vi "ScanCtrl_HRNoFP.vi"() -> ()   [LabVIEW 2020]
uses:
  <vilib>/event_ctls.llb/usereventprio.ctl
  C:/Users/MarcuLab/Desktop/V6 APD LV/V6 APD LV/Kinesis/Thorlabs.MotionControl.KCube.BrushlessMotorCLI.dll
  Kinesis/Thorlabs.MotionControl.KCube.BrushlessMotorCLI.dll
  C:/Users/MarcuLab/Desktop/V6 APD LV/V6 APD LV/Kinesis/ThorLabs.MotionControl.KCube.DCServoCLI.dll
  Kinesis/ThorLabs.MotionControl.KCube.DCServoCLI.dll
  C:/Users/MarcuLab/Desktop/V6 APD LV/V6 APD LV/Kinesis/Thorlabs.MotionControl.DeviceManagerCLI.dll
  Kinesis/Thorlabs.MotionControl.DeviceManagerCLI.dll
  C:/Users/MarcuLab/Desktop/V6 APD LV/V6 APD LV/Kinesis/Thorlabs.MotionControl.GenericMotorCLI.dll
  Kinesis/Thorlabs.MotionControl.GenericMotorCLI.dll
  <userlib>/_OpenG.lib/time/time.llb/openg_time.lvlib
panel:
  in  "GoToScanStart":bool
  in  "Home Button(fast)":bool
  out "Scan Progress":dbl(slide) scale=0.0..100.0
  in  "Jog Step (mm)":dbl=0.5
  in  "Down(Slow)":bool
  in  "Up(Slow)":bool
  in  "Down(Fast)":bool
  in  "Up(Fast)":bool
  out "SlowAxisStatus":T1
  out "SlowAxisInfo":T2
  out "FastAxisStatus":T1
  out "Current State":string
  out "FastAxisInfo":T3
  out "error out":errorcluster
  out "TriggerPara":T4
  out "Trigger1Polarity":i32(ring)=1 items=["TriggerHigh"=1, "TriggerLow"=2]
  out "Trigger1Mode":i32(ring) items=["Disabled"=0, "TrigIN_GPI"=1, "TrigIN_RelativeMove"=2, "TrigIN_AbsoluteMove"=3, "TrigIN_Homed"=4, "TrigIN_Stop"=5, "TrigOUT_GPO"=10, "TrigOUT_InMotion"=11, "TrigOUT_AtMaxVelocity"=12, "TrigOUT_AtPositionFwd"=13, "TrigOUT_AtPositionRev"=14, "TrigOUT_AtPositionBoth"=15, "TrigOut_AtFwdLimit"=16, "TrigOut_AtBwdLimit"=17, "TrigOut_AtLimit"=18]
  in  "acceleration (mm/s2)":dbl=4000.0
  out "ScanRoute":cluster{dbl[], dbl[]}(graph)
  out "# of lines":u32
  in  "Start Scan":bool
  in  "Comp Scan Para":bool
  out "X speed (mm/s)":dbl format="%.4g"
  in  "Laser Rate (Hz)":u16=2500
  in  "Y step size (um)":dbl=50.0
  in  "X step size (um)":dbl=10.0
  in  "Y scan distance (mm)":dbl=15.0
  in  "X scan distance (mm)":dbl=15.0
  out "Y0 Position(mm)":dbl format="%.4g"
  out "GetPositionCounter 2":i32
  out "X0 Position(mm)":dbl format="%.4g"
  out "GetPositionCounter":i32
  in  "SetScanStart":bool
  in  "SerialNumber(Slow)":string="27000986"
  in  "SerialNumber(Fast)":string="28252795"
  in  "Quit":bool
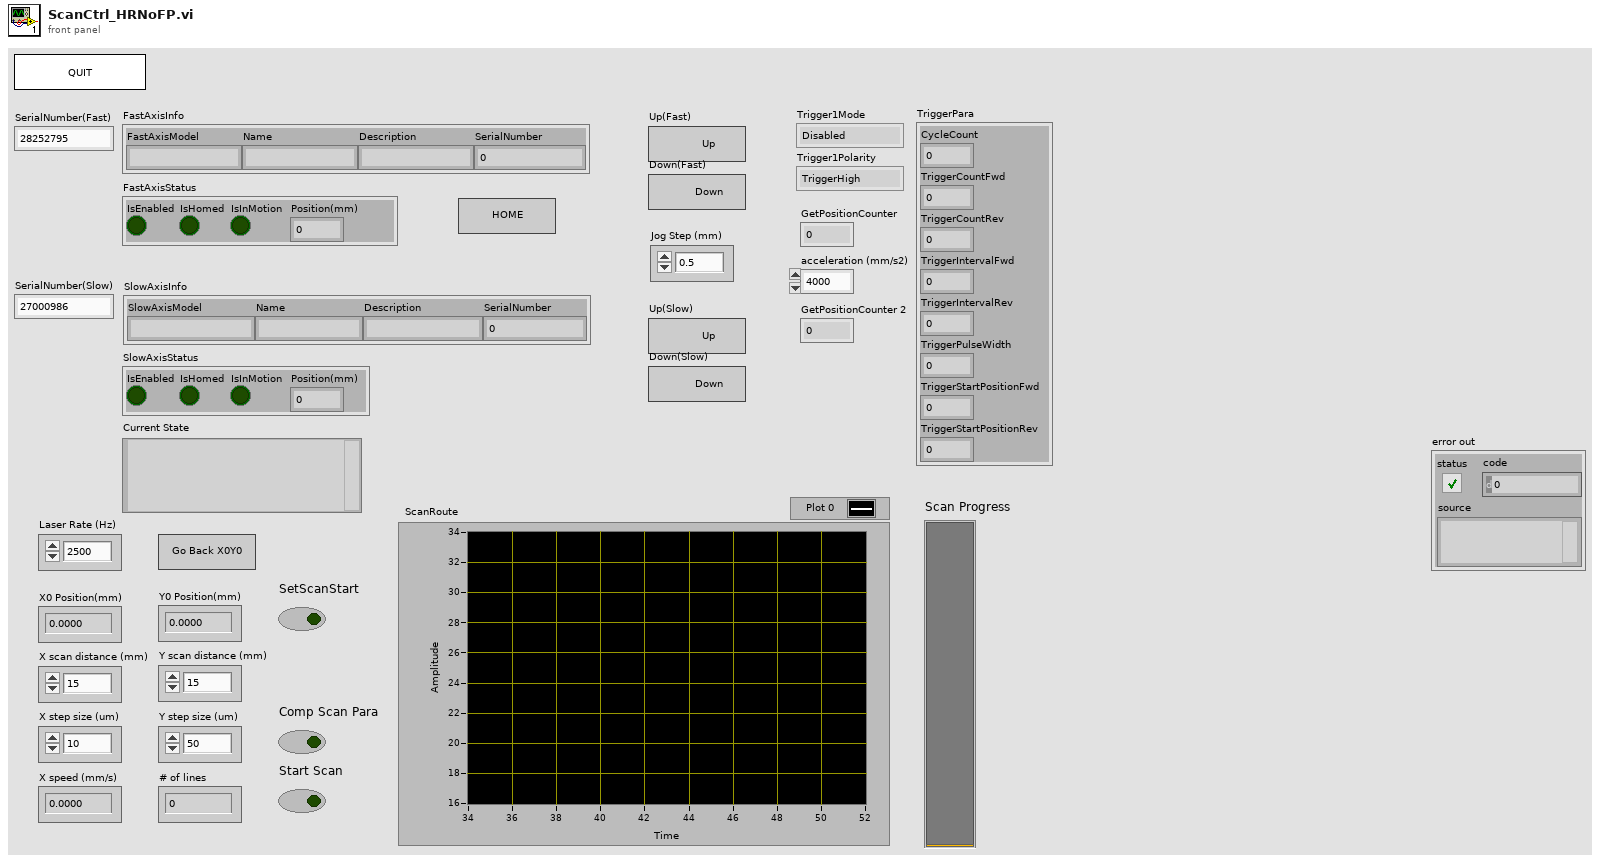
[diagram p1: front panel]
types:
  T1 = cluster{"IsEnabled":bool, "IsHomed":bool, "IsInMotion":bool, "Position(mm)":dbl}
  T2 = cluster{"SlowAxisModel":string, "Name":string, "Description":string, "SerialNumber":u32}
  T3 = cluster{"FastAxisModel":string, "Name":string, "Description":string, "SerialNumber":u32}
  T4 = cluster{"CycleCount":i32, "TriggerCountFwd":i32, "TriggerCountRev":i32, "TriggerIntervalFwd":dbl, "TriggerIntervalRev":dbl, "TriggerPulseWidth":i32, "TriggerStartPositionFwd":dbl, "TriggerStartPositionRev":dbl}
  T5 = cluster{"X":dbl[], "Y":dbl[], "Device(Fast)":refnum<k24>, "Device(Slow)":refnum<k24>}
  T6 = enum32{"Invalid", "Standard", "Closed", "Hidden", "Minimized", "Maximized"}
  T7 = enum32{"invalid app kind", "Development System", "Run Time System", "Student Edition", "Embedded LabVIEW", "Evaluation", "Custom"}
  T8 = typedef "usereventprio.ctl" = enum32{"high priority", "normal priority"}
  T9 = enum16{"open", "open or create", "create or replace", "create", "open (read-only)"}
  T10 = cluster{"Core":cluster{"Current VI Reference":refnum<vi>, "Close Panel on Exit?":bool}, "FastAxisSerial":string, "FastAxisModel":string, "SlowAxisSerial":string, "SlowAxisModel":string, "Device(Fast)":refnum<k24>, "Device(Slow)":refnum<k24>, "ScanRoute":cluster{dbl[], dbl[]}, "IsHomed(Fast)":bool, "IsHomed(Slow)":bool, "JogStep(mm)":dbl}
  T11 = cluster{"Current VI Reference":refnum<vi>, "Close Panel on Exit?":bool}
  T12 = cluster{"IsEnabled":bool, "IsHomed":bool, "IsInMotion":bool, "Position":dbl}
  T13 = cluster{"remote start event":refnum<user-event>, "remote stop event":refnum<user-event>}
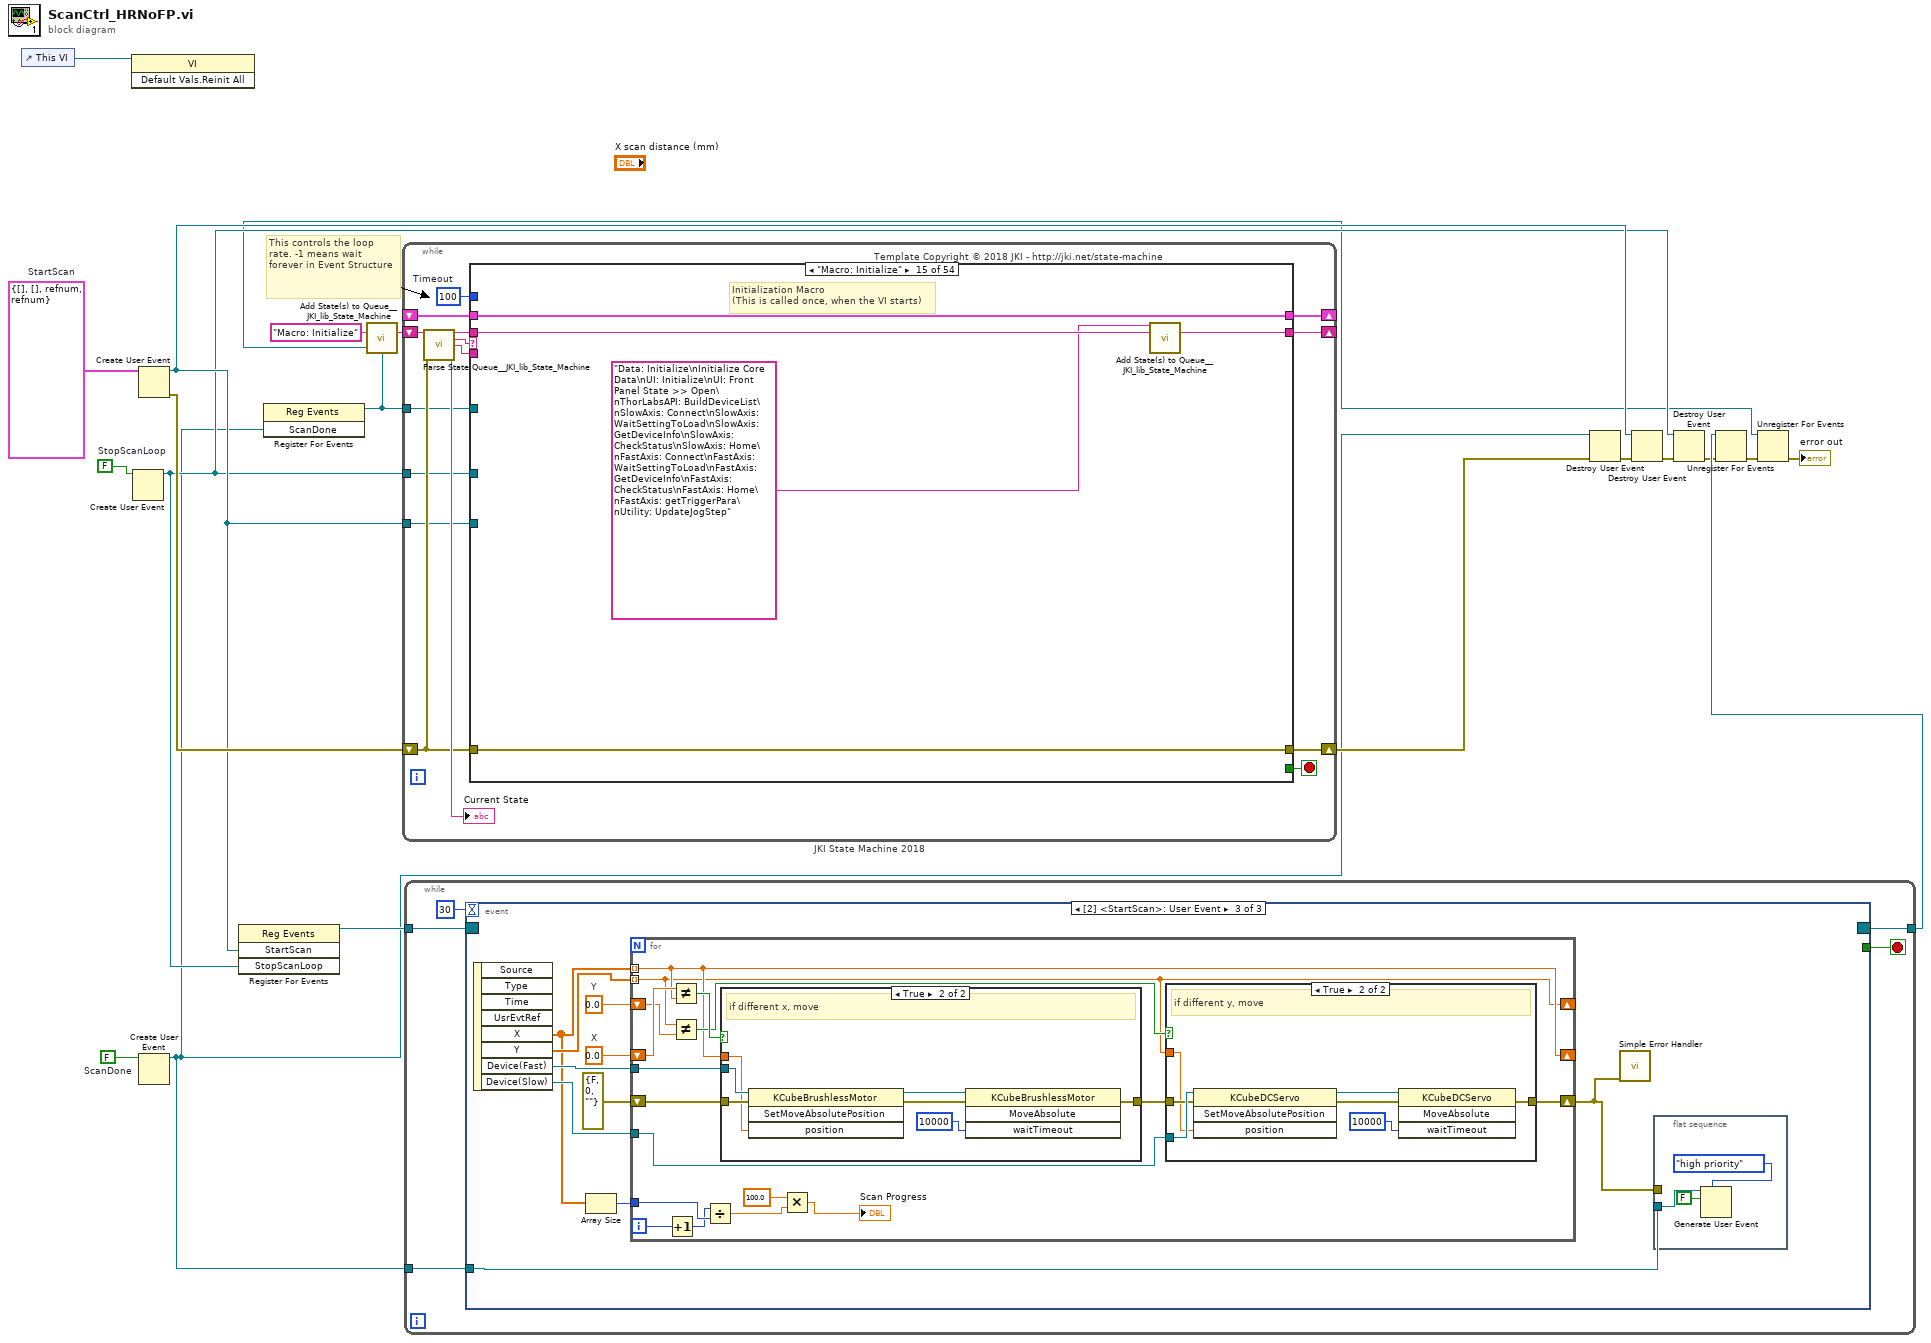
[diagram p0: block diagram]
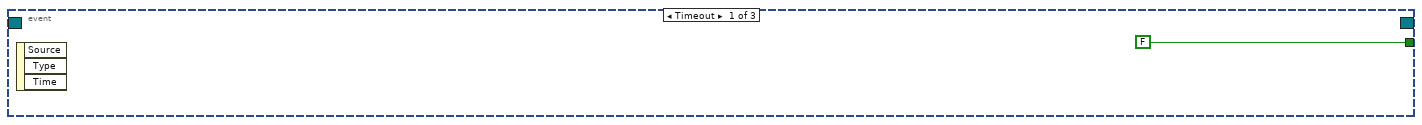
[diagram p2: hidden frame]
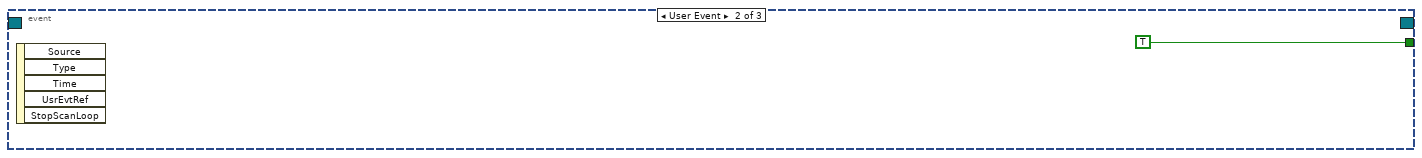
[diagram p3: hidden frame]
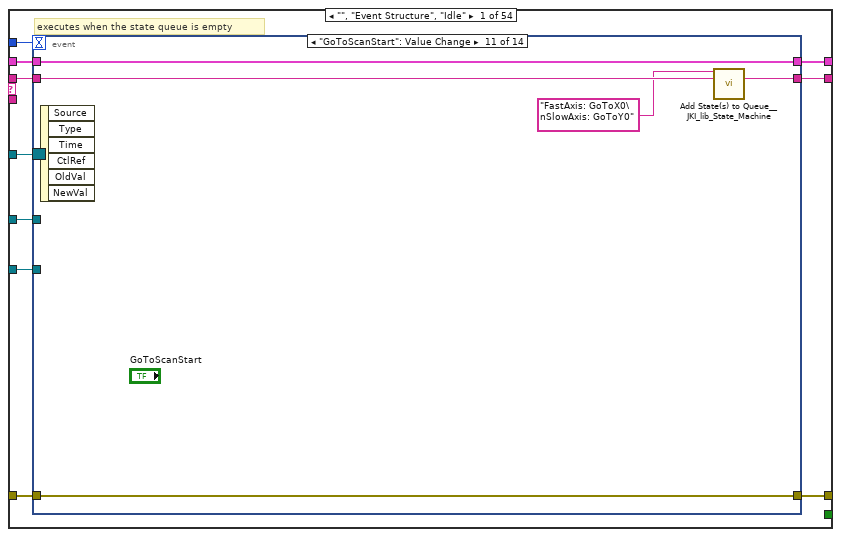
[diagram p6: hidden frame]
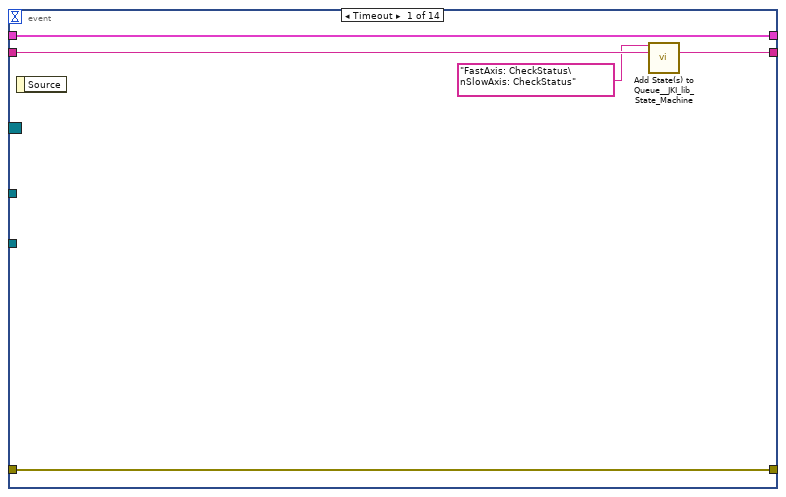
[diagram p7: hidden frame]
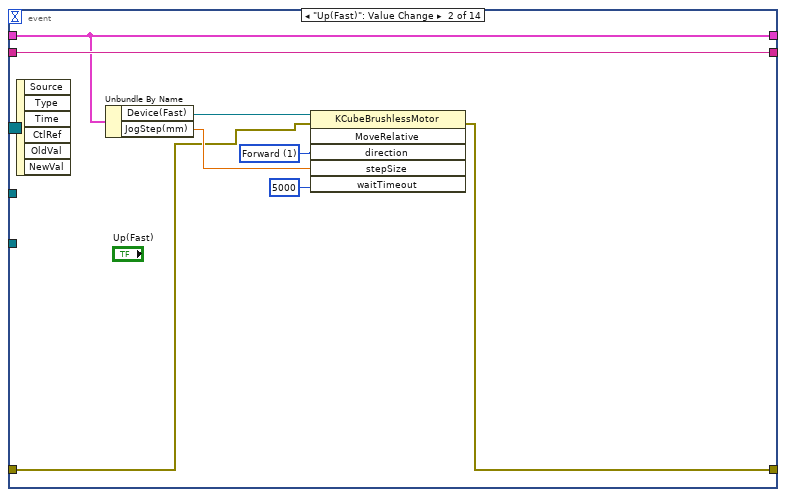
[diagram p8: hidden frame]
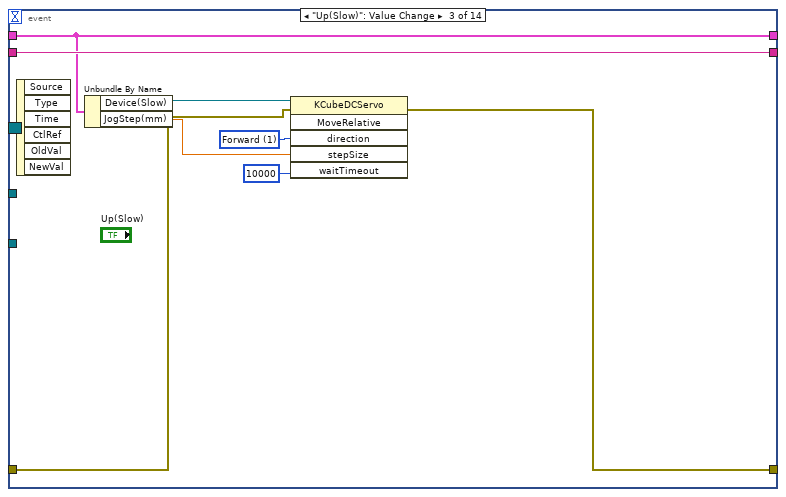
[diagram p9: hidden frame]
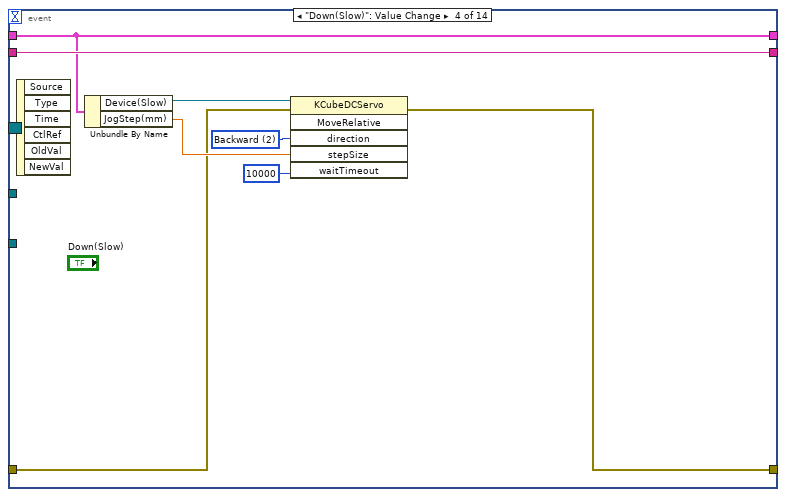
[diagram p10: hidden frame]
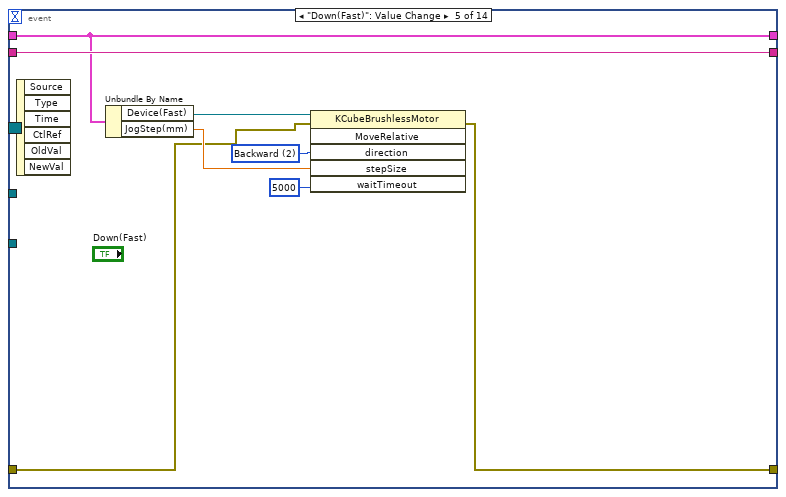
[diagram p11: hidden frame]
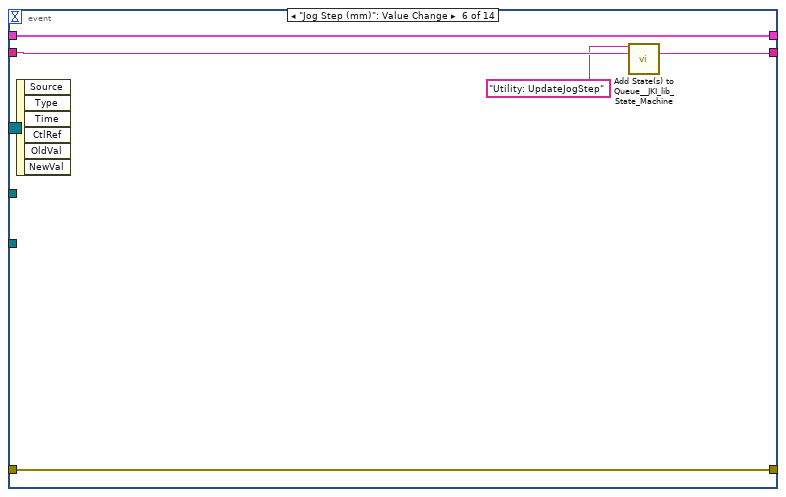
[diagram p12: hidden frame]
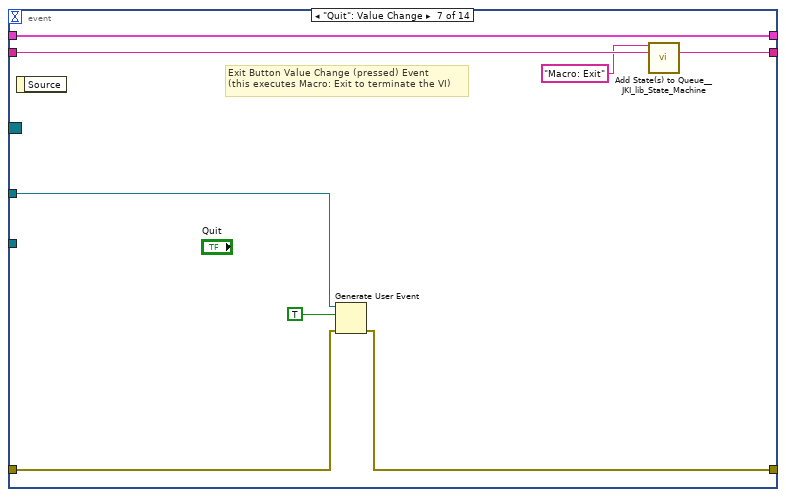
[diagram p13: hidden frame]
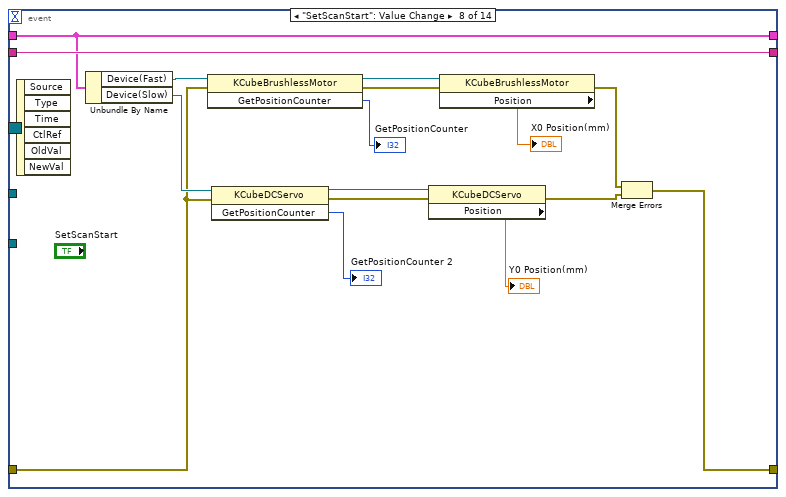
[diagram p14: hidden frame]
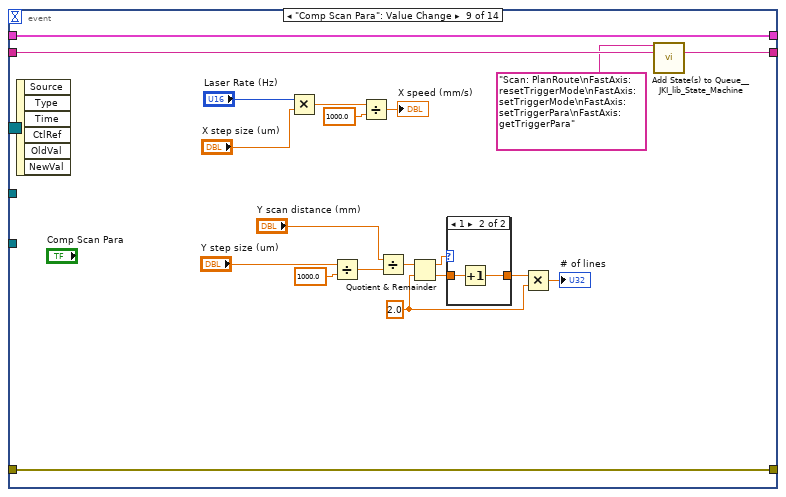
[diagram p15: hidden frame]
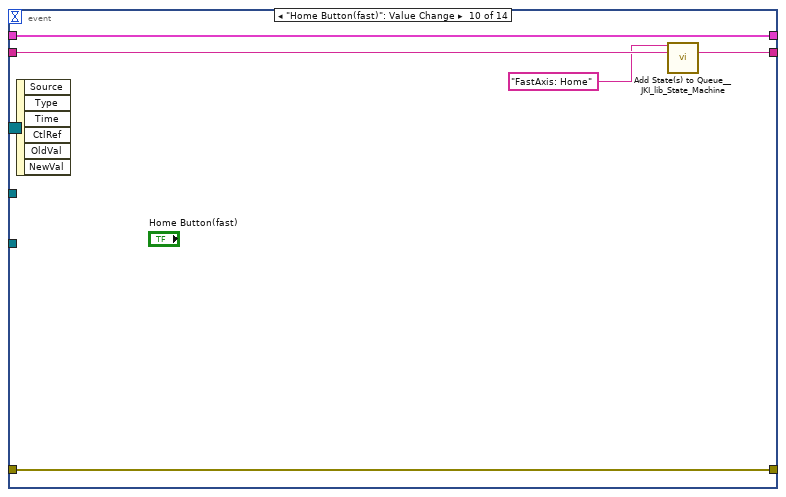
[diagram p17: hidden frame]
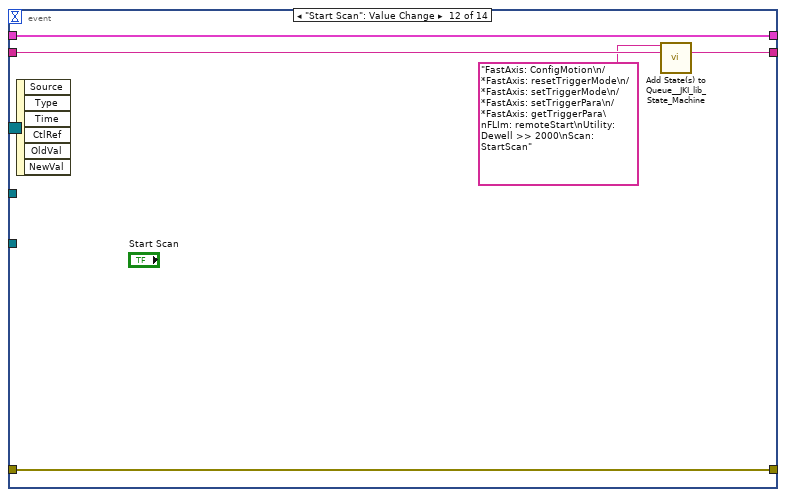
[diagram p18: hidden frame]
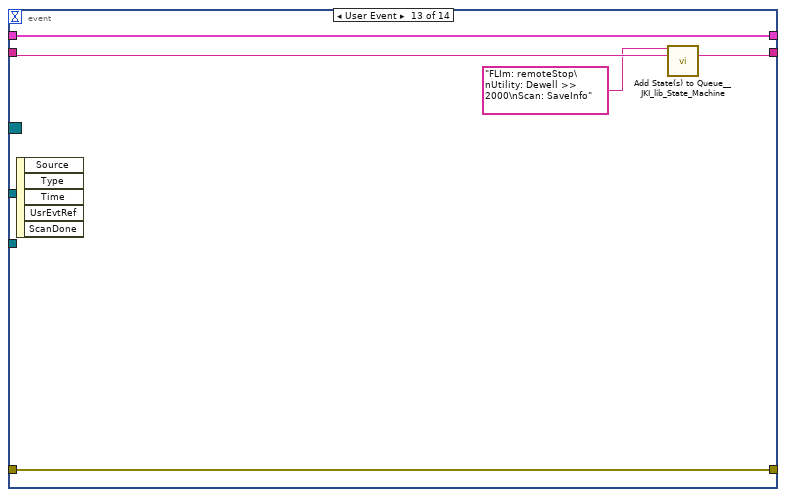
[diagram p19: hidden frame]
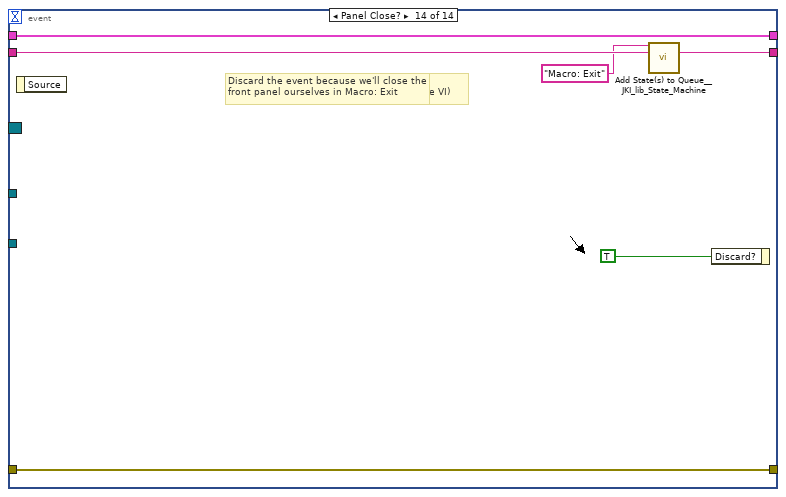
[diagram p20: hidden frame]
diagram:
  w13 = FALSE  # ScanDone
  w14 = T5 {"X"=[], "Y"=[], "Device(Fast)"=refnum, "Device(Slow)"=refnum}  # StartScan
  w15 = FALSE  # StopScanLoop
  # "This controls the loop rate. -1 means wait forever in Event Structure"
  n1 = control-ref of="This VI"() -> (w1:refnum<vi>)
  n2 = invoke class="VI" method="Default Vals.Reinit All"(reference=w1) -> ()  [unwired: 2 in, 3 out]
  n3 = Create User Event(user event datatype=w15) -> (user event=w10:refnum<user-event>)  [unwired: 1 in, 1 out]
  n4 = Create User Event(user event datatype=w14) -> (user event=w11:refnum<user-event>, error out=w16:errorcluster)  [unwired: 1 in]
  n5 = Create User Event(user event datatype=w13) -> (user event=w5:refnum<user-event>)  [unwired: 1 in, 1 out]
  n6 = register-events(w11, w10) -> (reference out=w17:refnum<event-registration>)  [unwired: 2 in, 1 out]
  n7 = register-events(w5) -> (reference out=w2:refnum<event-registration>)  [unwired: 2 in, 1 out]
  n8 = call <vilib>:"Add State(s) to Queue__JKI_lib_State_Machine.vi"("State(s) in (\"\")"="Macro: Initialize") -> ("States Out"=w19:string)  [unwired: 14 in]
  n9 = while "JKI State Machine 2018" {
    shift-right: [w26] -> _
    shift-left: _ -> [w25]
    shift-right: [w29] -> w6
    shift-left: w16 -> [w23]
    shift-right: [w28] -> _
    shift-left: w19 -> [w30]
    tunnel: w10 -> [w22]
    tunnel: w11 -> [w21]
    tunnel: w2 -> [w20]
    stop <- w27 stop-if-true
    w24 = 100  # Timeout
    # "Template Copyright © 2018 JKI - http://jki.net/state-machine"
    n10 = call <vilib>:"Parse State Queue__JKI_lib_State_Machine.vi"("State Queue"=w30, "Error In (no error)"=w23) -> ("Remaining States"=w32:string, "Current State"=w33:string, "Arguments"=w31:string)  [unwired: 11 in]
    "Current State" <- w33
    n11 = case shown="\"Macro: Initialize\"" w33 {
      selector: w33 -> [_ _ w163 _ _ _ _ _ _ _ _ _ _ _ _ _ _ _ _ _ _ _ _ _ _ _ _ _ _ _ _ _ _ _ _ _ _ _ _ _ _ _ _ _ _ _ _ _ _ _ _ _ _ _]
      tunnel: w32 -> [w43 w162 w167 w186 w192 w197 w201 w216 w222 w226 w230 w236 w247 w316 w321 w332 w336 w354 w360 w383 w396 w403 w425 w440 w455 w479 w485 w515 w523 w527 w545 w551 w570 w582 w589 w612 w616 w624 w628 w639 w685 w709 w713 w723 w733 w737 w743 w749 w754 w758 w764 w768 w772 w776]
      tunnel: w31 -> [_ _ _ _ _ _ _ _ _ _ _ w231 w241 _ _ _ _ _ _ _ _ _ _ _ _ _ _ _ _ _ _ _ _ _ _ _ _ _ _ _ _ _ _ _ _ _ w739 _ _ _ _ _ _ _]
      tunnel: w25 -> [w41 w159 w165 w179 w189 w195 w198 _ w217 w223 w228 w234 w243 w313 w318 w329 w333 w352 w358 w381 w391 w401 w423 w438 w453 w477 w483 w513 w521 w524 w544 w549 w568 w576 w587 w607 w613 w622 w625 w630 w675 w707 w710 w722 w731 w734 w740 w747 w750 w755 w762 w765 w769 w773]
      tunnel: [w40 w160 w169 w183 errorcluster {"status"=FALSE, "code"=0, "source"=""} ("error out") w194 w199 w213 w218 w224 w227 w232 w244 w314 w319 w330 w334 w341 w356 w377 w388 w398 w419 w429 w444 w459 w481 w508 w517 w525 w529 w547 w559 w580 w584 w605 w614 w621 w626 w638 w673 w687 w711 w715 w725 w735 w741 w745 w753 w756 w760 w766 w770 w774] -> w29
      tunnel: w23 -> [w39 w160 w168 w183 w188 w194 w199 w213 w219 w224 w227 w233 w245 w314 w319 w330 w334 w340 w355 w376 w387 w397 w418 w428 w443 w458 w480 w507 w517 w525 w530 w546 w558 w580 w583 w604 w614 w621 w626 w638 w672 w686 w711 w714 w724 w735 w741 w745 w753 w756 w759 w766 w770 w774]
      tunnel: [w42 w161 w166 w185 w191 w196 w200 w215 w221 w225 w229 w235 w246 w315 w320 w331 w335 w354 w359 w382 w396 w402 w424 w439 w454 w478 w484 w514 w522 w526 w545 w550 w569 w582 w588 w611 w615 w623 w627 w639 w684 w708 w712 w723 w732 w736 w742 w748 w754 w757 w763 w767 w771 w775] -> w28
      tunnel: [_ _ _ _ _ TRUE _ _ _ _ _ _ _ _ _ _ _ _ _ _ _ _ _ _ _ _ _ _ _ _ _ _ _ _ _ _ _ _ _ _ _ _ _ _ _ _ _ _ _ _ _ _ _ _] -> w27
      tunnel: [w38 w159 w165 w184 w189 w195 w198 w214 w217 w223 w228 w234 w243 w313 w318 w329 w333 w353 w358 w381 w392 w401 w423 w438 w453 w477 w483 w513 w521 w524 w543 w549 w568 w577 w587 w607 w613 w622 w625 w631 w675 w707 w710 w722 w731 w734 w740 w747 w751 w755 w762 w765 w769 w773] -> w26
      tunnel: w24 -> [w37 _ _ _ _ _ _ _ _ _ _ _ _ _ _ _ _ _ _ _ _ _ _ _ _ _ _ _ _ _ _ _ _ _ _ _ _ _ _ _ _ _ _ _ _ _ _ _ _ _ _ _ _ _]
      tunnel: w22 -> [w36 _ _ _ _ _ _ _ _ _ _ _ _ _ _ _ _ _ _ _ _ _ _ _ _ _ _ _ _ _ _ _ _ _ _ _ _ _ _ _ _ _ _ _ _ _ _ w746 _ _ _ _ _ _]
      tunnel: w21 -> [w35 _ _ _ _ _ _ _ _ _ _ _ _ _ _ _ _ _ _ _ _ _ _ _ _ _ _ _ _ _ _ _ _ _ _ _ _ _ _ _ w674 _ _ _ _ _ _ _ _ _ _ _ _ _]
      tunnel: w20 -> [w34 _ _ _ _ _ _ _ _ _ _ _ _ _ _ _ _ _ _ _ _ _ _ _ _ _ _ _ _ _ _ _ _ _ _ _ _ _ _ _ _ _ _ _ _ _ _ _ _ _ _ _ _ _]
      frame "", "Event Structure", "Idle" {
        # "executes when the state queue is empty"
        n12 = event shown="[10] \"GoToScanStart\": Value Change" {
          selector: w34 -> [_ _ _ _ _ _ _ _ _ _ _ _ _ _]
          dyn-events: _ -> [_ _ _ _ _ _ _ _ _ _ _ _ _ _]
          timeout: w37 -> [_ _ _ _ _ _ _ _ _ _ _ _ _ _]
          tunnel: w43 -> [w48 w56 w64 w72 w80 w83 w93 w109 w111 w135 w140 w145 w150 w158]
          tunnel: [w47 w56 w64 w72 w80 w82 w92 w109 w112 w134 w139 w146 w149 w157] -> w42
          tunnel: w41 -> [w45 w49 w57 w65 w73 w84 w91 w103 w123 w136 w141 w147 w151 w155]
          tunnel: [w46 w51 w59 w67 w75 w85 w87 w94 w124 w137 w142 w143 w152 w156] -> w40
          tunnel: w39 -> [w46 w50 w58 w66 w74 w85 w86 w101 w124 w137 w142 w143 w152 w156]
          tunnel: [w45 w49 w57 w65 w73 w84 w91 w103 w123 w136 w141 w147 w151 w155] -> w38
          tunnel: w36 -> [_ _ _ _ _ _ w89 _ _ _ _ _ _ _]
          tunnel: w35 -> [_ _ _ _ _ _ _ _ _ _ _ _ _ _]
          event Timeout {
            n13 = event-data() -> ()  [unwired: 1 in, 1 out]
            n14 = call <vilib>:"Add State(s) to Queue__JKI_lib_State_Machine.vi"("State(s) in Front (\"\")"="FastAxis: CheckStatus\nSlowAxis: CheckStatus" ("State(s) in Front (\"\")"), "State(s) in (\"\")"=w48) -> ("States Out"=w47:string)  [unwired: 13 in]
          }
          event "Up(Fast)": Value Change {
            w54 = 1 items=["Forward"=1, "Backward"=2] ("direction")
            n15 = event-data() -> ()  [unwired: 1 in, 6 out]
            n16 = Unbundle By Name(w49) -> ("Device(Fast)"=w55:refnum<k24>, "JogStep(mm)"=w53:dbl)
            n17 = invoke class="KCubeBrushlessMotor" method="MoveRelative"(reference=w55, error in=w50, "direction"=w54, "stepSize"=w53, "waitTimeout"=5000) -> (error out=w51:errorcluster)  [unwired: 1 in, 5 out]
          }
          event "Up(Slow)": Value Change {
            w62 = 1 items=["Forward"=1, "Backward"=2] ("direction")
            n18 = event-data() -> ()  [unwired: 1 in, 6 out]
            n19 = Unbundle By Name(w57) -> ("Device(Slow)"=w63:refnum<k24>, "JogStep(mm)"=w61:dbl)
            n20 = invoke class="KCubeDCServo" method="MoveRelative"(reference=w63, error in=w58, "direction"=w62, "stepSize"=w61, "waitTimeout"=10000) -> (error out=w59:errorcluster)  [unwired: 1 in, 5 out]
          }
          event "Down(Slow)": Value Change {
            w70 = 2 items=["Forward"=1, "Backward"=2] ("direction")
            n21 = event-data() -> ()  [unwired: 1 in, 6 out]
            n22 = Unbundle By Name(w65) -> ("Device(Slow)"=w71:refnum<k24>, "JogStep(mm)"=w69:dbl)
            n23 = invoke class="KCubeDCServo" method="MoveRelative"(reference=w71, error in=w66, "direction"=w70, "stepSize"=w69, "waitTimeout"=10000) -> (error out=w67:errorcluster)  [unwired: 1 in, 5 out]
          }
          event "Down(Fast)": Value Change {
            w78 = 2 items=["Forward"=1, "Backward"=2] ("direction")
            n24 = event-data() -> ()  [unwired: 1 in, 6 out]
            n25 = Unbundle By Name(w73) -> ("Device(Fast)"=w79:refnum<k24>, "JogStep(mm)"=w77:dbl)
            n26 = invoke class="KCubeBrushlessMotor" method="MoveRelative"(reference=w79, error in=w74, "direction"=w78, "stepSize"=w77, "waitTimeout"=5000) -> (error out=w75:errorcluster)  [unwired: 1 in, 5 out]
          }
          event "Jog Step (mm)": Value Change {
            n27 = event-data() -> ()  [unwired: 1 in, 6 out]
            n28 = call <vilib>:"Add State(s) to Queue__JKI_lib_State_Machine.vi"("State(s) in Front (\"\")"="Utility: UpdateJogStep" ("State(s) in Front (\"\")"), "State(s) in (\"\")"=w83) -> ("States Out"=w82:string)  [unwired: 13 in]
          }
          event "Quit": Value Change {
            # "Exit Button Value Change (pressed) Event\n(this executes Macro: Exit to terminate the VI)"
            n29 = event-data() -> ()  [unwired: 1 in, 1 out]
            n30 = Generate User Event(user event=w89, event data cluster=TRUE ("event data"), error in=w86) -> (error out=w87:errorcluster)  [unwired: 1 in, 1 out]
            n31 = call <vilib>:"Add State(s) to Queue__JKI_lib_State_Machine.vi"("State(s) in Front (\"\")"="Macro: Exit", "State(s) in (\"\")"=w93) -> ("States Out"=w92:string)  [unwired: 13 in]
          }
          event "SetScanStart": Value Change {
            n32 = event-data() -> ()  [unwired: 1 in, 6 out]
            n33 = Unbundle By Name(w103) -> ("Device(Fast)"=w108:refnum<k24>, "Device(Slow)"=w102:refnum<k24>)
            n34 = invoke class="KCubeBrushlessMotor" method="GetPositionCounter"(reference=w108, error in=w101) -> (reference out=w105:refnum<k24>, error out=w104:errorcluster, "GetPositionCounter"=→"GetPositionCounter":i32)  [unwired: 1 in]
            n35 = invoke class="KCubeDCServo" method="GetPositionCounter"(reference=w102, error in=w101) -> (reference out=w99:refnum<k24>, error out=w98:errorcluster, "GetPositionCounter"=→"GetPositionCounter 2":i32)  [unwired: 1 in]
            n36 = property class="KCubeDCServo"(reference=w99, error in=w98) -> (error out=w96:errorcluster, "Position"=→"Y0 Position(mm)":dbl)  [unwired: 1 out]
            n37 = property class="KCubeBrushlessMotor"(reference=w105, error in=w104) -> (error out=w95:errorcluster, "Position"=→"X0 Position(mm)":dbl)  [unwired: 1 out]
            n38 = Merge Errors(w95, w96) -> (w94:errorcluster)
          }
          event "Comp Scan Para": Value Change {
            w117 = 2.0 ("y")
            n39 = event-data() -> ()  [unwired: 1 in, 6 out]
            n40 = Multiply(x="Laser Rate (Hz)", y="X step size (um)") -> (x*y=w127:dbl)
            n41 = Divide(x="Y step size (um)", y=1000.0) -> (x/y=w120:dbl)
            n42 = Divide(x=w127, y=1000.0) -> (x/y=→"X speed (mm/s)":dbl)
            n43 = Divide(x="Y scan distance (mm)", y=w120) -> (x/y=w119:dbl)
            n44 = Quotient & Remainder(x=w119, y=w117) -> (x-y*floor(x/y)=w115:dbl, floor(x/y)=w114:dbl)
            n45 = case shown="1" w115 {
              tunnel: w114 -> [w130 w132]
              tunnel: [w130 w131] -> w113
              frame 0, Default {
              }
              frame 1 {
                n46 = Increment(x=w132) -> (x+1=w131:dbl)
              }
            }
            n47 = Multiply(x=w113, y=w117) -> (x*y=→"# of lines":dbl)
            n48 = call <vilib>:"Add State(s) to Queue__JKI_lib_State_Machine.vi"("State(s) in Front (\"\")"="Scan: PlanRoute\nFastAxis: resetTriggerMode\nFastAxis: setTriggerMode\nFastAxis: setTriggerPara\nFastAxis: getTriggerPara" ("State(s) in Front (\"\")"), "State(s) in (\"\")"=w111) -> ("States Out"=w112:string)  [unwired: 13 in]
          }
          event "Home Button(fast)": Value Change {
            n49 = event-data() -> ()  [unwired: 1 in, 6 out]
            n50 = call <vilib>:"Add State(s) to Queue__JKI_lib_State_Machine.vi"("State(s) in Front (\"\")"="FastAxis: Home" ("State(s) in Front (\"\")"), "State(s) in (\"\")"=w135) -> ("States Out"=w134:string)  [unwired: 13 in]
          }
          event "GoToScanStart": Value Change {
            n51 = event-data() -> ()  [unwired: 1 in, 6 out]
            n52 = call <vilib>:"Add State(s) to Queue__JKI_lib_State_Machine.vi"("State(s) in Front (\"\")"="FastAxis: GoToX0\nSlowAxis: GoToY0" ("State(s) in Front (\"\")"), "State(s) in (\"\")"=w140) -> ("States Out"=w139:string)  [unwired: 13 in]
          }
          event "Start Scan": Value Change {
            n53 = event-data() -> ()  [unwired: 1 in, 6 out]
            n54 = call <vilib>:"Add State(s) to Queue__JKI_lib_State_Machine.vi"("State(s) in Front (\"\")"="FastAxis: ConfigMotion\n/*FastAxis: resetTriggerMode\n/*FastAxis: setTriggerMode\n/*FastAxis: setTriggerPara\n/*FastAxis: getTriggerPara\nFLIm: remoteStart\nUtility: Dewell >> 2000\nScan: StartScan" ("State(s) in Front (\"\")"), "State(s) in (\"\")"=w145) -> ("States Out"=w146:string)  [unwired: 13 in]
          }
          event User Event {
            n55 = event-data() -> ()  [unwired: 1 in, 5 out]
            n56 = call <vilib>:"Add State(s) to Queue__JKI_lib_State_Machine.vi"("State(s) in Front (\"\")"="FLIm: remoteStop\nUtility: Dewell >> 2000\nScan: SaveInfo" ("State(s) in Front (\"\")"), "State(s) in (\"\")"=w150) -> ("States Out"=w149:string)  [unwired: 13 in]
          }
          event Panel Close? {
            # "Discard the event because we'll close the front panel ourselves in Macro: Exit"
            # "Close Panel button (pressed) Event\n(this executes Macro: Exit to terminate the VI)"
            n57 = event-data() -> ()  [unwired: 1 in, 1 out]
            n58 = call <vilib>:"Add State(s) to Queue__JKI_lib_State_Machine.vi"("State(s) in Front (\"\")"="Macro: Exit", "State(s) in (\"\")"=w158) -> ("States Out"=w157:string)  [unwired: 13 in]
            n59 = event-data("Discard?"=TRUE) -> ()  [unwired: 1 in, 1 out]
          }
        }
      }
      frame "---------- Core ----------" {
        # "Do not put any code in this frame.\n(it is a separator no-op)"
        n60 = call <vilib>:"Add State(s) to Queue__JKI_lib_State_Machine.vi"("State(s) in (\"\")"=w162) -> ("States Out"=w161:string)  [unwired: 14 in]
      }
      frame Default {
        w172 = 42 items=["No error", "Argument error", "Memory is full", "Out of zone", "End of file", "File already open", "Generic file I/O error", "File not found", "File permission error", "Disk is full", "Duplicate path", "Too many files open", "System feature not enabled", "Resource file not found", "Cannot add resource", "Resource not found", "Image not found", "Image memory error", "Pen does not exist", "Config type invalid", "Config token not found", "Config parse error", "Config memory error", "Bad external code format", "Bad external code offset", "External code not present", "Null window", "Destroy window error", "Null menu", "Print aborted", "Bad print record", "Print driver error", "Windows error during printing", "Memory error during printing", "Print dialog error", "Generic print error", "Invalid device refnum", "Device not found", "Device parameter error", "Device unit error", "Cannot open device", "Device call aborted", "Generic error", "Cancelled by user", "Object ID too low", "Object ID too high", "Object not in heap", "Unknown heap", "Unknown object (invalid DefProc)", "Unknown object (DefProc not in table)", "Message out of range", "Invalid (null) method", "Unknown message", "Manager call not supported", "Bad address", "Network operation in progress", "Network operation timed out", "Connection is busy", "Network attribute not supported", "Network error", "Address in use", "System out of memory", "Connection aborted", "Connection refused", "Not connected", "Already connected", "Connection closed", "Initialization error (interapplication manager)", "Bad occurrence", "Wait on unbound occurrence handler", "Occurrence queue overflow", "Datalog type conflict", "Unused", "Unrecognized type (interapplication manager)", "Memory corrupt", "Failed to make temporary DLL", "Old CIN version", "Drag socket not found", "Failed to load drop-object", "Failed to register OLE object", "Failed to release OLE object", "Format specifier type mismatch", "Unknown format specifier", "Too few format specifiers", "Too many format specifiers", "Scan failed", "Newer CIN version", "Error converting to variant", "Runtime menu error", "Password tampered", "Variant attribute not found", "Incompatible variant data type", "Event data is not available", "Event Store is not present", "Occurrence is not found", "Event Queue is not created", "Event info is not available", "Refnum passed is NULL", "Error retrieving Class GUID", "Error retrieving CoClass GUID", "Error retrieving TypeLib GUID.", "Bad built application magic bytes.", "Specific driver is different from the specific driver associated with the Logical Name.", "There is no session opened to the class driver.", "Max Error", "MAX - Error with config objects", "MAX - Error loading configuration", "MAX - Group not supported"]
        # "Current State"
        # "Do not delete, rename, or modify this frame.\n(this is used to capture unhandled states and typos)"
        # "Handle mistyped state name (developer tool)"
        n61 = Format Into String(format string="Software Exception: Unhandled State \"%s\"." ("message"), error in=w168, w163) -> (resulting string=w171:string, error out=w170:errorcluster)  [unwired: 1 in]
        n62 = call <vilib>:"Error Cluster From Error Code.vi"("show call chain? (False)"=TRUE, "error in (no error)"=w170, "error message (\"\")"=w171, "error code (0)"=w172) -> ("error out"=w169:errorcluster)  [unwired: 5 in]
        n63 = call <vilib>:"Add State(s) to Queue__JKI_lib_State_Machine.vi"("State(s) in (\"\")"=w167) -> ("States Out"=w166:string)  [unwired: 14 in]
      }
      frame "Initialize Core Data" {
        # "Do not delete, rename, or modify this frame.\n(this is used to determine panel behavior on exit)"
        # "originally closed?"
        # "exe?"
        # "If panel starts closed or is an EXE, then close it when we exit"
        n64 = property class="VI"() -> ("FP.State"=w176:T6)  [unwired: 2 in, 2 out]
        n65 = property class="App"() -> ("App.Kind"=w182:T7)  [unwired: 2 in, 2 out]
        n66 = control-ref of="Current VI Reference"() -> (w177:refnum<vi>)
        n67 = Equal?(x=w176, y=T6."Closed" ("Front Panel Window:State")) -> (x = y?=w174:bool)
        n68 = Equal?(x=w182, y=T7."Run Time System" ("Application:Kind")) -> (x = y?=w180:bool)
        n69 = Or(x=w174, y=w180) -> (x .or. y?=w178:bool)
        n70 = Bundle By Name(cluster=w179, "Core.Current VI Reference"=w177, "Core.Close Panel on Exit?"=w178) -> (w184:T10)
        n71 = call <vilib>:"Add State(s) to Queue__JKI_lib_State_Machine.vi"("State(s) in (\"\")"=w186) -> ("States Out"=w185:string)  [unwired: 14 in]
      }
      frame "Error Handler" {
        # "Unhandled Error -- Display it"
        # "Handle any errors here.\nYou can also output any states to clean-up after errors occur"
        # "Clear error"
        n72 = call <vilib>:"General Error Handler.vi"("error in (no error)"=w188) -> ()  [unwired: 10 in, 5 out]
        n73 = call <vilib>:"Add State(s) to Queue__JKI_lib_State_Machine.vi"("State(s) in Front (\"\")"="Macro: Exit\n/* Post Error States", "State(s) in (\"\")"=w192) -> ("States Out"=w191:string)  [unwired: 13 in]
      }
      frame "Exit" {
        # "Do not put any code in this frame.\n(No errors that occur here will be handled.)"
        n74 = call <vilib>:"Add State(s) to Queue__JKI_lib_State_Machine.vi"("State(s) in (\"\")"=w197) -> ("States Out"=w196:string)  [unwired: 14 in]
      }
      frame "---------- Data ----------" {
        # "Do not put any code in this frame.\n(It is a separator no-op. You can make a copy of this frame to create a new Data frame)"
        n75 = call <vilib>:"Add State(s) to Queue__JKI_lib_State_Machine.vi"("State(s) in (\"\")"=w201) -> ("States Out"=w200:string)  [unwired: 14 in]
      }
      frame "Data: Initialize" {
        w202 = 0.0  # JogStep(mm)
        w203 = "MTS50-Z8"  # SlowAxisModel
        w204 = FALSE  # IsHomed(Slow)
        w205 = FALSE  # IsHomed(Fast)
        w206 = "DDS100"  # FastAxisModel
        w207 = cluster{dbl[], dbl[]} {[], []}  # ScanRoute
        w208 = refnum<k24> refnum  # Device(Slow)
        w209 = refnum<k24> refnum  # Device(Fast)
        w210 = ""  # SlowAxisSerial
        w211 = T11 {"Current VI Reference"=refnum, "Close Panel on Exit?"=FALSE}  # Core
        w212 = ""  # FastAxisSerial
        # "do not delete - used by framework"
        # "Data names and types of shift register data are defined by this bundle."
        # "Initialize the shift-register data, here.\n(data names are defined by what you wire into the bundle function)"
        n76 = Bundle("Core"=w211, "FastAxisSerial"=w212, "FastAxisModel"=w206, "SlowAxisSerial"=w210, "SlowAxisModel"=w203, "Device(Fast)"=w209, "Device(Slow)"=w208, "ScanRoute"=w207, "IsHomed(Fast)"=w205, "IsHomed(Slow)"=w204, "JogStep(mm)"=w202) -> (w214:T10)  [unwired: 1 in]
        n77 = call <vilib>:"Add State(s) to Queue__JKI_lib_State_Machine.vi"("State(s) in (\"\")"=w216) -> ("States Out"=w215:string)  [unwired: 14 in]
      }
      frame "Data: Cleanup" {
        # "Cleanup any data and references, here.\n(this is called automatically, by the Macro: Exit)"
        n78 = Unbundle By Name(w217) -> ("Core.Current VI Reference"=w220:refnum<vi>)
        n79 = Close Reference(reference=w220, error in (no error)=w219) -> (error out=w218:errorcluster)
        n80 = call <vilib>:"Add State(s) to Queue__JKI_lib_State_Machine.vi"("State(s) in (\"\")"=w222) -> ("States Out"=w221:string)  [unwired: 14 in]
      }
      frame "---------- UI ----------" {
        # "Do not put any code in this frame.\n(It is a separator no-op. You can make a copy of this frame to create a new UI frame)"
        n81 = call <vilib>:"Add State(s) to Queue__JKI_lib_State_Machine.vi"("State(s) in (\"\")"=w226) -> ("States Out"=w225:string)  [unwired: 14 in]
      }
      frame "UI: Initialize" {
        # "Initialize the User Interface, here.\n(this is called automatically, by the Macro: Init)"
        n82 = call <vilib>:"Add State(s) to Queue__JKI_lib_State_Machine.vi"("State(s) in (\"\")"=w230) -> ("States Out"=w229:string)  [unwired: 14 in]
      }
      frame "UI: Cursor Set" {
        # "Argument"
        # "Set and Unset Cursor Busy.\n(Usage: \"UI: Cursor Set >> Busy|Idle\")"
        n83 = case shown="\"Idle\", Default" w231 {
          tunnel: w233 -> [w238 w240]
          tunnel: [w237 w239] -> w232
          frame "Idle", Default {
            n84 = call <vilib>:"Unset Busy.vi"("error in (no error)"=w238) -> ("error out"=w237:errorcluster)  [unwired: 10 in]
          }
          frame "Busy" {
            n85 = call <vilib>:"Set Busy.vi"("error in (no error)"=w240) -> ("error out"=w239:errorcluster)  [unwired: 9 in, 1 out]
          }
        }
        n86 = call <vilib>:"Add State(s) to Queue__JKI_lib_State_Machine.vi"("State(s) in (\"\")"=w236) -> ("States Out"=w235:string)  [unwired: 14 in]
      }
      frame "UI: Front Panel State" {
        # "Argument"
        # "Set Front Panel Open or Closed\n(Usage: \"UI: Front Panel State >> Open|Close\")"
        n87 = Unbundle By Name(w243) -> ("Core.Current VI Reference"=w242:refnum<vi>)
        n88 = case shown="\"Minimize\", \"Minimized\"" w241 {
          tunnel: w245 -> [w253 w268 w279 w292 w305]
          tunnel: [w255 w269 w281 w294 w307] -> w244
          tunnel: w242 -> [w254 w266 w280 w293 w306]
          frame "Open", "Standard", Default {
            w248 = T6."Standard" ("State")
            n89 = property class="VI"(reference=w254, error in=w253) -> (reference out=w251:refnum<vi>, error out=w252:errorcluster, "FP.State"=w250:T6)
            n90 = Not Equal?(x=w250, y=w248) -> (x != y?=w249:bool)
            n91 = case shown="True" w249 {
              tunnel: [w259 w261] -> w255
              tunnel: w252 -> [w258 w261]
              tunnel: w251 -> [w257 _]
              tunnel: w248 -> [w256 _]
              frame True {
                n92 = invoke class="VI" method="FP.Open"(reference=w257, error in=w258, "Activate"=TRUE, "State"=w256) -> (error out=w259:errorcluster)  [unwired: 1 in, 4 out]
              }
              frame False {
              }
            }
          }
          frame "Close", "Closed" {
            n93 = property class="VI"(reference=w266, error in=w268) -> (reference out=w265:refnum<vi>, error out=w267:errorcluster, "FP.State"=w263:T6)
            n94 = Not Equal?(x=w263, y=T6."Closed" ("Front Panel Window:State")) -> (x != y?=w262:bool)
            n95 = case shown="True" w262 {
              tunnel: [w270 w273] -> w269
              tunnel: w267 -> [w270 w272]
              tunnel: w265 -> [_ w271]
              frame False {
              }
              frame True {
                n96 = invoke class="VI" method="FP.Close"(reference=w271, error in=w272) -> (error out=w273:errorcluster)  [unwired: 1 in, 2 out]
              }
            }
          }
          frame "Hidden", "Hide" {
            w274 = T6."Hidden" ("State")
            n97 = property class="VI"(reference=w280, error in=w279) -> (reference out=w277:refnum<vi>, error out=w278:errorcluster, "FP.State"=w276:T6)
            n98 = Not Equal?(x=w276, y=w274) -> (x != y?=w275:bool)
            n99 = case shown="True" w275 {
              tunnel: [w285 w286] -> w281
              tunnel: w278 -> [w284 w286]
              tunnel: w277 -> [w283 _]
              tunnel: w274 -> [w282 _]
              frame True {
                n100 = invoke class="VI" method="FP.Open"(reference=w283, error in=w284, "State"=w282) -> (error out=w285:errorcluster)  [unwired: 2 in, 4 out]
              }
              frame False {
              }
            }
          }
          frame "Minimize", "Minimized" {
            w287 = T6."Minimized" ("State")
            n101 = property class="VI"(reference=w293, error in=w292) -> (reference out=w290:refnum<vi>, error out=w291:errorcluster, "FP.State"=w289:T6)
            n102 = Not Equal?(x=w289, y=w287) -> (x != y?=w288:bool)
            n103 = case shown="True" w288 {
              tunnel: [w298 w299] -> w294
              tunnel: w291 -> [w297 w299]
              tunnel: w290 -> [w296 _]
              tunnel: w287 -> [w295 _]
              frame True {
                n104 = invoke class="VI" method="FP.Open"(reference=w296, error in=w297, "State"=w295) -> (error out=w298:errorcluster)  [unwired: 2 in, 4 out]
              }
              frame False {
              }
            }
          }
          frame "Maximize", "Maximized" {
            w300 = T6."Maximized" ("State")
            n105 = property class="VI"(reference=w306, error in=w305) -> (reference out=w303:refnum<vi>, error out=w304:errorcluster, "FP.State"=w302:T6)
            n106 = Not Equal?(x=w302, y=w300) -> (x != y?=w301:bool)
            n107 = case shown="True" w301 {
              tunnel: [w311 w312] -> w307
              tunnel: w304 -> [w310 w312]
              tunnel: w303 -> [w309 _]
              tunnel: w300 -> [w308 _]
              frame True {
                n108 = invoke class="VI" method="FP.Open"(reference=w309, error in=w310, "State"=w308) -> (error out=w311:errorcluster)  [unwired: 2 in, 4 out]
              }
              frame False {
              }
            }
          }
        }
        n109 = call <vilib>:"Add State(s) to Queue__JKI_lib_State_Machine.vi"("State(s) in (\"\")"=w247) -> ("States Out"=w246:string)  [unwired: 14 in]
      }
      frame "---------- Macro ----------" {
        # "Do not put any code in this frame.\n(It is a separator no-op. You can make a copy of this frame to create a new Macro frame)"
        n110 = call <vilib>:"Add State(s) to Queue__JKI_lib_State_Machine.vi"("State(s) in (\"\")"=w316) -> ("States Out"=w315:string)  [unwired: 14 in]
      }
      frame "Macro: Initialize" {
        # "Initialization Macro\n(This is called once, when the VI starts)"
        n111 = call <vilib>:"Add State(s) to Queue__JKI_lib_State_Machine.vi"("State(s) in Front (\"\")"="Data: Initialize\nInitialize Core Data\nUI: Initialize\nUI: Front Panel State >> Open\nThorLabsAPI: BuildDeviceList\nSlowAxis: Connect\nSlowAxis: WaitSettingToLoad\nSlowAxis: GetDeviceInfo\nSlowAxis: CheckStatus\nSlowAxis: Home\nFastAxis: Connect\nFastAxis: WaitSettingToLoad\nFastAxis: GetDeviceInfo\nFastAxis: CheckStatus\nFastAxis: Home\nFastAxis: getTriggerPara\nUtility: UpdateJogStep", "State(s) in (\"\")"=w321) -> ("States Out"=w320:string)  [unwired: 13 in]
      }
      frame "Macro: Exit" {
        # "Exit Macro\n(This is called once, when the VI exits)"
        n112 = Unbundle By Name(w329) -> ("Core.Close Panel on Exit?"=w328:bool)
        n113 = Select(t="UI: Front Panel State >> Close", s=w328, f="") -> (s? t:f=w325:string)
        n114 = call <vilib>:"Add State(s) to Queue__JKI_lib_State_Machine.vi"("State(s) in Front (\"\")"="FastAxis: Close\nSlowAxis: Close" ("State(s) in Front (\"\")"), "State(s) in (\"\")"=w325, "State(s) at Back (\"\")"="Utility: StopScanLoop\nData: Cleanup\nExit") -> ("States Out"=w323:string)  [unwired: 12 in]
        n115 = call <vilib>:"Add State(s) to Queue__JKI_lib_State_Machine.vi"("State(s) in Front (\"\")"=w323, "State(s) in (\"\")"=w332) -> ("States Out"=w331:string)  [unwired: 13 in]
      }
      frame "---------- FastAxis ----------" {
        # "Template Separator\n(You can make a copy of, or modify, this frame)"
        n116 = call <vilib>:"Add State(s) to Queue__JKI_lib_State_Machine.vi"("State(s) in (\"\")"=w336) -> ("States Out"=w335:string)  [unwired: 14 in]
      }
      frame "FastAxis: Connect" {
        w346 = 3 items=["UseDeviceSettings"=1, "UseFileSettings"=2, "UseConfiguredSettings"=3] ("startupSettingsMode")
        # "wait for 1s or the next function will throw error"
        # "Open Fast Axis\n(You can make a copy of, or modify, this frame)"
        n117 = invoke class="KCubeBrushlessMotor" method="CreateKCubeBrushlessMotor"(reference=refnum<k24> refnum, error in=w340, "serialNo"="SerialNumber(Fast)") -> (error out=w350:errorcluster, "CreateKCubeBrushlessMotor"=w349:refnum<k24>)  [unwired: 1 in, 2 out]
        n118 = invoke class="KCubeBrushlessMotor" method="Connect"(reference=w349, error in=w350, "serialNo"="SerialNumber(Fast)") -> (reference out=w348:refnum<k24>, error out=w339:errorcluster)  [unwired: 1 in, 2 out]
        n119 = call <userlib>:"Wait (ms)__ogtk.vi"("error in (no error)"=w339, "milliseconds to wait"=u32 1000) -> ("error out"=w338:errorcluster)  [unwired: 8 in, 1 out]
        n120 = invoke class="KCubeBrushlessMotor" method="LoadMotorConfiguration"(reference=w348, error in=w338, "serialNo"="SerialNumber(Fast)", "startupSettingsMode"=w346) -> (reference out=w344:refnum<k24>, error out=w345:errorcluster)  [unwired: 1 in, 3 out]
        n121 = invoke class="KCubeBrushlessMotor" method="StartPolling"(reference=w344, error in=w345, "ms"=250) -> (reference out=w342:refnum<k24>, error out=w341:errorcluster)  [unwired: 1 in, 2 out]
        n122 = Bundle By Name(cluster=w352, "FastAxisSerial"="SerialNumber(Fast)", "Device(Fast)"=w342) -> (w353:T10)
      }
      frame "FastAxis: WaitSettingToLoad" {
        # "wait for device setting to finish loading\n(You can make a copy of, or modify, this frame)"
        n123 = Unbundle By Name(w358) -> ("Device(Fast)"=w357:refnum<k24>)
        n124 = while {
          tunnel: w357 -> [w366]
          shift-right: [w364] -> w356
          shift-left: w355 -> [w361]
          stop <- w362 stop-if-true
          n125 = invoke class="KCubeBrushlessMotor" method="IsSettingsInitialized"(reference=w366, error in=w361) -> (error out=w364:errorcluster, "IsSettingsInitialized"=w363:bool)  [unwired: 1 in, 1 out]
          n126 = Wait (ms)(milliseconds to wait=u32 100) -> ()  [unwired: 1 out]
          n127 = Or(x=w364, y=w363) -> (x .or. y?=w362:bool)
        }
        n128 = call <vilib>:"Add State(s) to Queue__JKI_lib_State_Machine.vi"("State(s) in (\"\")"=w360) -> ("States Out"=w359:string)  [unwired: 14 in]
      }
      frame "FastAxis: GetDeviceInfo" {
        # "Template Separator\n(You can make a copy of, or modify, this frame)"
        n129 = Unbundle By Name(w381) -> ("Device(Fast)"=w380:refnum<k24>, "FastAxisModel"=w372:string)
        n130 = invoke class="KCubeBrushlessMotor" method="GetDeviceInfo"(reference=w380, error in=w376) -> (reference out=w367:refnum<k24>, error out=w379:errorcluster, "GetDeviceInfo"=w378:refnum<k24>)  [unwired: 1 in]
        n131 = invoke class="KCubeBrushlessMotor" method="GetVelocityParams"(reference=w367, "maxVelocity"=0.0, "acceleration"=0.0) -> ("acceleration"=w370:dbl)  [unwired: 2 in, 4 out]
        n132 = property class="DeviceInfo"(reference=w378, error in=w379) -> (error out=w377:errorcluster, "Name"=w375:string, "Description"=w374:string, "SerialNumber"=w373:u32)  [unwired: 1 out]
        n133 = Bundle("FastAxisModel"=w372, "Name"=w375, "Description"=w374, "SerialNumber"=w373) -> (→"FastAxisInfo":T3)  [unwired: 1 in]
        n134 = local write "acceleration (mm/s2)"(w370) -> ()
        n135 = call <vilib>:"Add State(s) to Queue__JKI_lib_State_Machine.vi"("State(s) in (\"\")"=w383) -> ("States Out"=w382:string)  [unwired: 14 in]
      }
      frame "FastAxis: CheckStatus" {
        # "check whether stahe is homed, if not home stage\n(You can make a copy of, or modify, this frame)"
        n136 = Unbundle By Name(w391) -> ("Device(Fast)"=w395:refnum<k24>)
        n137 = property class="KCubeBrushlessMotor"(reference=w395, error in=w387) -> (error out=w389:errorcluster, "Status"=w394:refnum<k24>, "Position"=w393:dbl)  [unwired: 1 out]
        n138 = property class="StatusBase"(reference=w394, error in=w389) -> (error out=w388:errorcluster, "IsEnabled"=w390:bool, "IsHomed"=w386:bool, "IsInMotion"=w385:bool)  [unwired: 1 out]
        n139 = Bundle("IsEnabled"=w390, "IsHomed"=w386, "IsInMotion"=w385, "Position"=w393) -> (→"FastAxisStatus":T12)  [unwired: 1 in]
        n140 = Bundle By Name(cluster=w391, "IsHomed(Fast)"=w386) -> (w392:T10)
      }
      frame "FastAxis: Home" {
        # "Home stage\n(You can make a copy of, or modify, this frame)"
        n141 = Unbundle By Name(w401) -> ("IsHomed(Fast)"=w400:bool, "Device(Fast)"=w399:refnum<k24>)
        n142 = case shown="False" w400 {
          tunnel: w399 -> [w406 _]
          tunnel: w397 -> [w405 w417]
          tunnel: [w404 w417] -> w398
          frame False {
            # "if not homed, home"
            n143 = stacked-sequence {
              seq-local: [_ w410 _] -> [_ _ w413]
              tunnel: w406 -> [_ w412 w416]
              tunnel: w405 -> [_ w411 _]
              tunnel: [_ _ w414] -> w404
              frame #0 {
                # "show dialog"
                n144 = One Button Dialog(message="Fast Axis will home!\nPlease make sure it is cleared of any object", button name ("OK")="Confirm!") -> ()  [unwired: 1 out]
              }
              frame #1 {
                # "enable device"
                n145 = invoke class="KCubeBrushlessMotor" method="EnableDevice"(reference=w412, error in=w411) -> (error out=w410:errorcluster)  [unwired: 1 in, 2 out]
                n146 = Wait (ms)(milliseconds to wait=u32 1000) -> ()  [unwired: 1 out]
              }
              frame #2 {
                # "home stage"
                n147 = invoke class="KCubeBrushlessMotor" method="Home"(reference=w416, error in=w413, "waitTimeout"=20000) -> (error out=w414:errorcluster)  [unwired: 1 in, 3 out]
              }
            }
          }
          frame True {
            # "if homed, do nothing"
          }
        }
        n148 = call <vilib>:"Add State(s) to Queue__JKI_lib_State_Machine.vi"("State(s) in (\"\")"=w403) -> ("States Out"=w402:string)  [unwired: 14 in]
      }
      frame "FastAxis: ConfigMotion" {
        # "Config fast axis speed\n(You can make a copy of, or modify, this frame)"
        n149 = local read "X speed (mm/s)"() -> (w420:dbl)
        n150 = Unbundle By Name(w423) -> ("Device(Fast)"=w422:refnum<k24>)
        n151 = invoke class="KCubeBrushlessMotor" method="SetVelocityParams"(reference=w422, error in=w418, "maxVelocity"=w420, "acceleration"="acceleration (mm/s2)") -> (error out=w419:errorcluster)  [unwired: 1 in, 4 out]
        n152 = call <vilib>:"Add State(s) to Queue__JKI_lib_State_Machine.vi"("State(s) in (\"\")"=w425) -> ("States Out"=w424:string)  [unwired: 14 in]
      }
      frame "FastAxis: setTriggerMode" {
        w426 = 1 items=["TriggerHigh"=1, "TriggerLow"=2] ("Trigger2Polarity")
        w427 = 0 items=["Disabled"=0, "TrigIN_GPI"=1, "TrigIN_RelativeMove"=2, "TrigIN_AbsoluteMove"=3, "TrigIN_Homed"=4, "TrigIN_Stop"=5, "TrigOUT_GPO"=10, "TrigOUT_InMotion"=11, "TrigOUT_AtMaxVelocity"=12, "TrigOUT_AtPositionFwd"=13, "TrigOUT_AtPositionRev"=14, "TrigOUT_AtPositionBoth"=15, "TrigOut_AtFwdLimit"=16, "TrigOut_AtBwdLimit"=17, "TrigOut_AtLimit"=18] ("Trigger2Mode")
        w433 = 1 items=["TriggerHigh"=1, "TriggerLow"=2] ("Trigger1Polarity")
        w434 = 15 items=["Disabled"=0, "TrigIN_GPI"=1, "TrigIN_RelativeMove"=2, "TrigIN_AbsoluteMove"=3, "TrigIN_Homed"=4, "TrigIN_Stop"=5, "TrigOUT_GPO"=10, "TrigOUT_InMotion"=11, "TrigOUT_AtMaxVelocity"=12, "TrigOUT_AtPositionFwd"=13, "TrigOUT_AtPositionRev"=14, "TrigOUT_AtPositionBoth"=15, "TrigOut_AtFwdLimit"=16, "TrigOut_AtBwdLimit"=17, "TrigOut_AtLimit"=18] ("Trigger1Mode")
        # "Config trigger out \n(You can make a copy of, or modify, this frame)"
        n153 = Unbundle By Name(w438) -> ("Device(Fast)"=w437:refnum<k24>)
        n154 = invoke class="KCubeBrushlessMotor" method="GetTriggerConfigParams"(reference=w437, error in=w428) -> (reference out=w436:refnum<k24>, error out=w431:errorcluster, "GetTriggerConfigParams"=w435:refnum<k24>)  [unwired: 1 in]
        n155 = property class="KCubeTriggerConfigParams"(reference=w435, error in=w431, "Trigger1Mode"=w434, "Trigger1Polarity"=w433, "Trigger2Mode"=w427, "Trigger2Polarity"=w426) -> (reference out=w432:refnum<k24>, error out=w430:errorcluster)
        n156 = invoke class="KCubeBrushlessMotor" method="SetTriggerConfigParams"(reference=w436, error in=w430, "triggerConfigParameters"=w432) -> (error out=w429:errorcluster)  [unwired: 1 in, 3 out]
        n157 = call <vilib>:"Add State(s) to Queue__JKI_lib_State_Machine.vi"("State(s) in (\"\")"=w440) -> ("States Out"=w439:string)  [unwired: 14 in]
      }
      frame "FastAxis: resetTriggerMode" {
        w441 = 1 items=["TriggerHigh"=1, "TriggerLow"=2] ("Trigger2Polarity")
        w442 = 0 items=["Disabled"=0, "TrigIN_GPI"=1, "TrigIN_RelativeMove"=2, "TrigIN_AbsoluteMove"=3, "TrigIN_Homed"=4, "TrigIN_Stop"=5, "TrigOUT_GPO"=10, "TrigOUT_InMotion"=11, "TrigOUT_AtMaxVelocity"=12, "TrigOUT_AtPositionFwd"=13, "TrigOUT_AtPositionRev"=14, "TrigOUT_AtPositionBoth"=15, "TrigOut_AtFwdLimit"=16, "TrigOut_AtBwdLimit"=17, "TrigOut_AtLimit"=18] ("Trigger2Mode")
        w448 = 1 items=["TriggerHigh"=1, "TriggerLow"=2] ("Trigger1Polarity")
        w449 = 0 items=["Disabled"=0, "TrigIN_GPI"=1, "TrigIN_RelativeMove"=2, "TrigIN_AbsoluteMove"=3, "TrigIN_Homed"=4, "TrigIN_Stop"=5, "TrigOUT_GPO"=10, "TrigOUT_InMotion"=11, "TrigOUT_AtMaxVelocity"=12, "TrigOUT_AtPositionFwd"=13, "TrigOUT_AtPositionRev"=14, "TrigOUT_AtPositionBoth"=15, "TrigOut_AtFwdLimit"=16, "TrigOut_AtBwdLimit"=17, "TrigOut_AtLimit"=18] ("Trigger1Mode")
        # "reset trigger mode\n(You can make a copy of, or modify, this frame)"
        n158 = Unbundle By Name(w453) -> ("Device(Fast)"=w452:refnum<k24>)
        n159 = invoke class="KCubeBrushlessMotor" method="GetTriggerConfigParams"(reference=w452, error in=w443) -> (reference out=w451:refnum<k24>, error out=w446:errorcluster, "GetTriggerConfigParams"=w450:refnum<k24>)  [unwired: 1 in]
        n160 = property class="KCubeTriggerConfigParams"(reference=w450, error in=w446, "Trigger1Mode"=w449, "Trigger1Polarity"=w448, "Trigger2Mode"=w442, "Trigger2Polarity"=w441) -> (reference out=w447:refnum<k24>, error out=w445:errorcluster)
        n161 = invoke class="KCubeBrushlessMotor" method="SetTriggerConfigParams"(reference=w451, error in=w445, "triggerConfigParameters"=w447) -> (error out=w444:errorcluster)  [unwired: 1 in, 3 out]
        n162 = call <vilib>:"Add State(s) to Queue__JKI_lib_State_Machine.vi"("State(s) in (\"\")"=w455) -> ("States Out"=w454:string)  [unwired: 14 in]
      }
      frame "FastAxis: setTriggerPara" {
        # "set trigger parameter\n(You can make a copy of, or modify, this frame)"
        n163 = Unbundle By Name(w477) -> ("Device(Fast)"=w476:refnum<k24>)
        n164 = local read "X step size (um)"() -> (w469:dbl)
        n165 = local read "X scan distance (mm)"() -> (w464:dbl)
        n166 = local read "X0 Position(mm)"() -> (w465:dbl)
        n167 = local read "# of lines"() -> (w473:u32)
        n168 = invoke class="KCubeBrushlessMotor" method="GetTriggerParamsParams"(reference=w476, error in=w458) -> (reference out=w462:refnum<k24>, error out=w474:errorcluster, "GetTriggerParamsParams"=w475:refnum<k24>)  [unwired: 1 in]
        n169 = Divide(x=w469, y=1000.0) -> (x/y=w467:dbl)
        n170 = Divide(x=w473, y=u32 2) -> (x/y=w457:dbl)
        n171 = Add(x=w465, y=w467) -> (x+y=w466:dbl)
        n172 = Divide(x=w464, y=w467) -> (x/y=w470:dbl)
        n173 = Add(x=w465, y=w464) -> (x+y=w463:dbl)
        n174 = Decrement(x=w457) -> (x-1=w456:dbl)
        n175 = property class="KCubeTriggerParamsParameters"(reference=w475, error in=w474, "CycleCount"=w456, "TriggerCountFwd"=w470, "TriggerCountRev"=w470, "TriggerIntervalFwd"=w467, "TriggerIntervalRev"=w467, "TriggerPulseWidth"=50, "TriggerStartPositionFwd"=w466, "TriggerStartPositionRev"=w463) -> (reference out=w460:refnum<k24>, error out=w461:errorcluster)
        n176 = invoke class="KCubeBrushlessMotor" method="SetTriggerParamsParams"(reference=w462, error in=w461, "triggerParamsParameters"=w460) -> (error out=w459:errorcluster)  [unwired: 1 in, 3 out]
        n177 = call <vilib>:"Add State(s) to Queue__JKI_lib_State_Machine.vi"("State(s) in (\"\")"=w479) -> ("States Out"=w478:string)  [unwired: 14 in]
      }
      frame "FastAxis: getTriggerPara" {
        # "Get Current Trigger Setting\n(You can make a copy of, or modify, this frame)"
        n178 = Unbundle By Name(w483) -> ("Device(Fast)"=w482:refnum<k24>)
        n179 = stacked-sequence {
          tunnel: w482 -> [w491 w505]
          tunnel: w480 -> [w490 w504]
          tunnel: [_ w492] -> w481
          frame #0 {
            # "get tigger configuration"
            n180 = invoke class="KCubeBrushlessMotor" method="GetTriggerConfigParams"(reference=w491, error in=w490) -> (error out=w488:errorcluster, "GetTriggerConfigParams"=w489:refnum<k24>)  [unwired: 1 in, 1 out]
            n181 = property class="KCubeTriggerConfigParams" props=["Trigger1Mode", "Trigger1Polarity", "Trigger2Mode", "Trigger2Polarity"](reference=w489, error in=w488) -> ("Trigger1Mode"=→"Trigger1Mode":i32, "Trigger1Polarity"=→"Trigger1Polarity":i32)  [unwired: 4 out]
          }
          frame #1 {
            # "get trigger parameter"
            n182 = invoke class="KCubeBrushlessMotor" method="GetTriggerParamsParams"(reference=w505, error in=w504) -> (error out=w502:errorcluster, "GetTriggerParamsParams"=w503:refnum<k24>)  [unwired: 1 in, 1 out]
            n183 = property class="KCubeTriggerParamsParameters"(reference=w503, error in=w502) -> (error out=w492:errorcluster, "CycleCount"=w501:i32, "TriggerCountFwd"=w500:i32, "TriggerCountRev"=w499:i32, "TriggerIntervalFwd"=w498:dbl, "TriggerIntervalRev"=w497:dbl, "TriggerPulseWidth"=w496:i32, "TriggerStartPositionFwd"=w495:dbl, "TriggerStartPositionRev"=w494:dbl)  [unwired: 1 out]
            n184 = Bundle("CycleCount"=w501, "TriggerCountFwd"=w500, "TriggerCountRev"=w499, "TriggerIntervalFwd"=w498, "TriggerIntervalRev"=w497, "TriggerPulseWidth"=w496, "TriggerStartPositionFwd"=w495, "TriggerStartPositionRev"=w494) -> (→"TriggerPara":T4)  [unwired: 1 in]
          }
        }
        n185 = call <vilib>:"Add State(s) to Queue__JKI_lib_State_Machine.vi"("State(s) in (\"\")"=w485) -> ("States Out"=w484:string)  [unwired: 14 in]
      }
      frame "FastAxis: GoToX0" {
        # "Template Separator\n(You can make a copy of, or modify, this frame)"
        n186 = Unbundle By Name(w513) -> ("Device(Fast)"=w512:refnum<k24>)
        n187 = local read "X0 Position(mm)"() -> (w506:dbl)
        n188 = invoke class="KCubeBrushlessMotor" method="SetMoveAbsolutePosition"(reference=w512, error in=w507, "position"=w506) -> (reference out=w511:refnum<k24>, error out=w510:errorcluster)  [unwired: 1 in, 2 out]
        n189 = invoke class="KCubeBrushlessMotor" method="MoveAbsolute"(reference=w511, error in=w510, "waitTimeout"=10000) -> (error out=w508:errorcluster)  [unwired: 1 in, 3 out]
        n190 = call <vilib>:"Add State(s) to Queue__JKI_lib_State_Machine.vi"("State(s) in (\"\")"=w515) -> ("States Out"=w514:string)  [unwired: 14 in]
      }
      frame "FastAxis: Close" {
        # "Template Separator\n(You can make a copy of, or modify, this frame)"
        n191 = Unbundle By Name(w521) -> ("Device(Fast)"=w519:refnum<k24>)
        n192 = invoke class="KCubeBrushlessMotor" method="StopPolling"(reference=w519) -> (reference out=w518:refnum<k24>, error out=w516:errorcluster)  [unwired: 2 in, 1 out]
        n193 = invoke class="KCubeBrushlessMotor" method="Disconnect"(reference=w518, error in=w516) -> (error out=w520:errorcluster)  [unwired: 1 in, 2 out]
        n194 = call <vilib>:"Simple Error Handler.vi"("error in (no error)"=w520) -> ()  [unwired: 4 in, 5 out]
        n195 = call <vilib>:"Add State(s) to Queue__JKI_lib_State_Machine.vi"("State(s) in (\"\")"=w523) -> ("States Out"=w522:string)  [unwired: 14 in]
      }
      frame "---------- SlowAxis ----------" {
        # "Template Separator\n(You can make a copy of, or modify, this frame)"
        n196 = call <vilib>:"Add State(s) to Queue__JKI_lib_State_Machine.vi"("State(s) in (\"\")"=w527) -> ("States Out"=w526:string)  [unwired: 14 in]
      }
      frame "SlowAxis: Connect" {
        w540 = 3 items=["UseDeviceSettings"=1, "UseFileSettings"=2, "UseConfiguredSettings"=3] ("startupSettingsMode")
        # "Template Separator\n(You can make a copy of, or modify, this frame)"
        n197 = invoke class="KCubeDCServo" method="CreateKCubeDCServo"(reference=refnum<k24> refnum ("target class"), error in=w530, "serialNo"="SerialNumber(Slow)") -> (error out=w541:errorcluster, "CreateKCubeDCServo"=w528:refnum<k24>)  [unwired: 1 in, 2 out]
        n198 = invoke class="KCubeDCServo" method="Connect"(reference=w528, error in=w541, "device"="SerialNumber(Slow)") -> (reference out=w538:refnum<k24>, error out=w537:errorcluster)  [unwired: 1 in, 2 out]
        n199 = call <userlib>:"Wait (ms)__ogtk.vi"("error in (no error)"=w537, "milliseconds to wait"=u32 500) -> ("error out"=w536:errorcluster)  [unwired: 8 in, 1 out]
        n200 = invoke class="KCubeDCServo" method="LoadMotorConfiguration"(reference=w538, error in=w536, "serialNo"="SerialNumber(Slow)", "startupSettingsMode"=w540) -> (reference out=w534:refnum<k24>, error out=w533:errorcluster)  [unwired: 1 in, 3 out]
        n201 = invoke class="KCubeDCServo" method="StartPolling"(reference=w534, error in=w533, "ms"=250) -> (reference out=w531:refnum<k24>, error out=w529:errorcluster)  [unwired: 1 in, 2 out]
        n202 = Bundle By Name(cluster=w544, "SlowAxisSerial"="SerialNumber(Slow)", "Device(Slow)"=w531) -> (w543:T10)
      }
      frame "SlowAxis: WaitSettingToLoad" {
        # "Template Separator\n(You can make a copy of, or modify, this frame)"
        n203 = Unbundle By Name(w549) -> ("Device(Slow)"=w548:refnum<k24>)
        n204 = while {
          tunnel: w548 -> [w557]
          shift-right: [w554] -> w547
          shift-left: w546 -> [w555]
          stop <- w552 stop-if-true
          n205 = invoke class="KCubeDCServo" method="IsSettingsInitialized"(reference=w557, error in=w555) -> (error out=w554:errorcluster, "IsSettingsInitialized"=w553:bool)  [unwired: 1 in, 1 out]
          n206 = Wait (ms)(milliseconds to wait=u32 100) -> ()  [unwired: 1 out]
          n207 = Or(x=w554, y=w553) -> (x .or. y?=w552:bool)
        }
        n208 = call <vilib>:"Add State(s) to Queue__JKI_lib_State_Machine.vi"("State(s) in (\"\")"=w551) -> ("States Out"=w550:string)  [unwired: 14 in]
      }
      frame "SlowAxis: GetDeviceInfo" {
        # "Template Separator\n(You can make a copy of, or modify, this frame)"
        n209 = Unbundle By Name(w568) -> ("SlowAxisModel"=w564:string, "Device(Slow)"=w565:refnum<k24>)
        n210 = invoke class="KCubeDCServo" method="GetDeviceInfo"(reference=w565, error in=w558) -> (error out=w566:errorcluster, "GetDeviceInfo"=w567:refnum<k24>)  [unwired: 1 in, 1 out]
        n211 = property class="DeviceInfo"(reference=w567, error in=w566) -> (error out=w559:errorcluster, "Name"=w563:string, "Description"=w562:string, "SerialNumber"=w561:u32)  [unwired: 1 out]
        n212 = Bundle("SlowAxisModel"=w564, "Name"=w563, "Description"=w562, "SerialNumber"=w561) -> (→"SlowAxisInfo":T2)  [unwired: 1 in]
        n213 = call <vilib>:"Add State(s) to Queue__JKI_lib_State_Machine.vi"("State(s) in (\"\")"=w570) -> ("States Out"=w569:string)  [unwired: 14 in]
      }
      frame "SlowAxis: CheckStatus" {
        # "Template Separator\n(You can make a copy of, or modify, this frame)"
        n214 = Unbundle By Name(w576) -> ("Device(Slow)"=w581:refnum<k24>)
        n215 = property class="KCubeDCServo"(reference=w581, error in=w580) -> (error out=w578:errorcluster, "Status"=w579:refnum<k24>, "Position"=w572:dbl)  [unwired: 1 out]
        n216 = property class="StatusBase"(reference=w579, error in=w578) -> ("IsEnabled"=w575:bool, "IsHomed"=w574:bool, "IsInMotion"=w573:bool)  [unwired: 2 out]
        n217 = Bundle("IsEnabled"=w575, "IsHomed"=w574, "IsInMotion"=w573, "Position"=w572) -> (→"SlowAxisStatus":T12)  [unwired: 1 in]
        n218 = Bundle By Name(cluster=w576, "IsHomed(Slow)"=w574) -> (w577:T10)
      }
      frame "SlowAxis: Home" {
        # "Template Separator\n(You can make a copy of, or modify, this frame)"
        n219 = Unbundle By Name(w587) -> ("IsHomed(Slow)"=w586:bool, "Device(Slow)"=w585:refnum<k24>)
        n220 = case shown="False" w586 {
          tunnel: w585 -> [w597 _]
          tunnel: [w591 w602] -> w584
          tunnel: w583 -> [w590 w602]
          frame False {
            n221 = flat-sequence {
              tunnel: [w599] -> w598
              tunnel: w590 -> [w599]
              frame #0 {
                n222 = One Button Dialog(message="Slow Axis will home.\nPlease clear all obstacles!", button name ("OK")="Confirm!") -> ()  [unwired: 1 out]
              }
            }
            n223 = invoke class="KCubeDCServo" method="EnableDevice"(reference=w597, error in=w598) -> (reference out=w594:refnum<k24>, error out=w596:errorcluster)  [unwired: 1 in, 1 out]
            n224 = call <userlib>:"Wait (ms)__ogtk.vi"("error in (no error)"=w596, "milliseconds to wait"=u32 500) -> ("error out"=w593:errorcluster)  [unwired: 8 in, 1 out]
            n225 = invoke class="KCubeDCServo" method="Home"(reference=w594, error in=w593, "waitTimeout"=60000) -> (error out=w591:errorcluster)  [unwired: 1 in, 3 out]
          }
          frame True {
          }
        }
        n226 = call <vilib>:"Add State(s) to Queue__JKI_lib_State_Machine.vi"("State(s) in (\"\")"=w589) -> ("States Out"=w588:string)  [unwired: 14 in]
      }
      frame "SlowAxis: GoToY0" {
        # "Template Separator\n(You can make a copy of, or modify, this frame)"
        n227 = local read "Y0 Position(mm)"() -> (w603:dbl)
        n228 = Unbundle By Name(w607) -> ("Device(Slow)"=w606:refnum<k24>)
        n229 = invoke class="KCubeDCServo" method="SetMoveAbsolutePosition"(reference=w606, error in=w604, "position"=w603) -> (reference out=w610:refnum<k24>, error out=w609:errorcluster)  [unwired: 1 in, 2 out]
        n230 = invoke class="KCubeDCServo" method="MoveAbsolute"(reference=w610, error in=w609, "waitTimeout"=10000) -> (error out=w605:errorcluster)  [unwired: 1 in, 3 out]
        n231 = call <vilib>:"Add State(s) to Queue__JKI_lib_State_Machine.vi"("State(s) in (\"\")"=w612) -> ("States Out"=w611:string)  [unwired: 14 in]
      }
      frame "SlowAxis: ConfigMotion" {
        # "Template Separator\n(You can make a copy of, or modify, this frame)"
        n232 = call <vilib>:"Add State(s) to Queue__JKI_lib_State_Machine.vi"("State(s) in (\"\")"=w616) -> ("States Out"=w615:string)  [unwired: 14 in]
      }
      frame "SlowAxis: Close" {
        # "Template Separator\n(You can make a copy of, or modify, this frame)"
        n233 = Unbundle By Name(w622) -> ("Device(Slow)"=w620:refnum<k24>)
        n234 = invoke class="KCubeDCServo" method="StopPolling"(reference=w620) -> (reference out=w619:refnum<k24>, error out=w618:errorcluster)  [unwired: 2 in, 1 out]
        n235 = invoke class="KCubeDCServo" method="Disconnect"(reference=w619, error in=w618) -> (error out=w617:errorcluster)  [unwired: 1 in, 2 out]
        n236 = call <vilib>:"Simple Error Handler.vi"("error in (no error)"=w617) -> ()  [unwired: 4 in, 5 out]
        n237 = call <vilib>:"Add State(s) to Queue__JKI_lib_State_Machine.vi"("State(s) in (\"\")"=w624) -> ("States Out"=w623:string)  [unwired: 14 in]
      }
      frame "---------- Scan ----------" {
        # "Template Separator\n(You can make a copy of, or modify, this frame)"
        n238 = call <vilib>:"Add State(s) to Queue__JKI_lib_State_Machine.vi"("State(s) in (\"\")"=w628) -> ("States Out"=w627:string)  [unwired: 14 in]
      }
      frame "Scan: PlanRoute" {
        # "Compute Scan Route\n(You can make a copy of, or modify, this frame)"
        n239 = local read "Y0 Position(mm)"() -> (w634:dbl)
        n240 = local read "# of lines"() -> (w637:u32)
        n241 = Multiply(x=w637, y=u32 2) -> (x*y=w635:u32)
        n242 = for {
          N: w635 -> [_]
          tunnel: [w647] -> w633 mode=indexing
          shift-right: [w643] -> _
          shift-left: w634 -> [w645]
          tunnel: [w643] -> w632 mode=indexing
          i -> [w642]
          n243 = Quotient & Remainder(x=w642, y=2) -> (x-y*floor(x/y)=w646:i32)  [unwired: 1 out]
          n244 = Quotient & Remainder(x=w642, y=4) -> (x-y*floor(x/y)=w640:i32)  [unwired: 1 out]
          n245 = case "X case" shown="0, 3, Default" w640 {
            tunnel: [w656 w668] -> w647
            frame 0, 3, Default {
              n246 = local read "X step size (um)"() -> (w661:dbl)
              n247 = local read "X0 Position(mm)"() -> (w662:dbl)
              n248 = Divide(x=w661, y=1000.0) -> (x/y=w659:dbl)
              n249 = Multiply(x=w659, y=10.0) -> (x*y=w657:dbl)
              n250 = Subtract(x=w662, y=w657) -> (x-y=w656:dbl)
            }
            frame 1, 2 {
              n251 = local read "X step size (um)"() -> (w667:dbl)
              n252 = local read "X scan distance (mm)"() -> (w670:dbl)
              n253 = local read "X0 Position(mm)"() -> (w671:dbl)
              n254 = Divide(x=w667, y=1000.0) -> (x/y=w665:dbl)
              n255 = Add(x=w671, y=w670) -> (x+y=w669:dbl)
              n256 = Multiply(x=w665, y=10.0) -> (x*y=w663:dbl)
              n257 = Add(x=w669, y=w663) -> (x+y=w668:dbl)
            }
          }
          n258 = case shown="0, Default" w646 {
            tunnel: [w649 0.0 ("x")] -> w644
            tunnel: w642 -> [w652 _]
            frame 0, Default {
              n259 = local read "Y step size (um)"() -> (w654:dbl)
              n260 = Sign(1:w652) -> (0:w651:i32)
              n261 = Divide(x=w654, y=1000.0) -> (x/y=w650:dbl)
              n262 = Multiply(x=w650, y=w651) -> (x*y=w649:dbl)
            }
            frame 1 {
            }
          }
          n263 = Add(x=w644, y=w645) -> (x+y=w643:dbl)
        }
        n264 = Bundle(w633, w632) -> (w629:cluster{dbl[], dbl[]})  [unwired: 1 in]
        "ScanRoute" <- w629
        n265 = Bundle By Name(cluster=w630, "ScanRoute"=w629) -> (w631:T10)
      }
      frame "Scan: StartScan" {
        w677 = T5 {"X"=[], "Y"=[], "Device(Fast)"=refnum, "Device(Slow)"=refnum}  # StartScan
        # "Generate user event to start scan\n(You can make a copy of, or modify, this frame)"
        n266 = Unbundle By Name(w675) -> ("ScanRoute"=w683:cluster{dbl[], dbl[]}, "Device(Fast)"=w680:refnum<k24>, "Device(Slow)"=w679:refnum<k24>)
        n267 = Unbundle(w683) -> (w682:dbl[], w681:dbl[])
        n268 = Bundle By Name(cluster=w677, "X"=w682, "Y"=w681, "Device(Fast)"=w680, "Device(Slow)"=w679) -> (w678:T5)
        n269 = Generate User Event(priority (normal)=usereventprio."high priority", user event=w674, event data cluster=w678, error in=w672) -> (error out=w673:errorcluster)  [unwired: 1 out]
        n270 = call <vilib>:"Add State(s) to Queue__JKI_lib_State_Machine.vi"("State(s) in (\"\")"=w685) -> ("States Out"=w684:string)  [unwired: 14 in]
      }
      frame "Scan: SaveInfo" {
        # "save scan information to encoder TDMS\n(You can make a copy of, or modify, this frame)"
        n271 = call "EncoderTDMS_Path.vi"("error in (no error)"=w686, "Operation (Read)"=enum16{"Write", "Read"}."Read") -> ("error out"=w704:errorcluster, "Path Out"=w705:path)  [unwired: 8 in]
        n272 = TDMS Open(8:w704, 10:T9."open" ("operation (0:open)"), 11:w705) -> (0:w701:errorcluster, 3:w702:refnum<k34>)  [unwired: 4 in]
        n273 = local read "# of lines"() -> (w691:u32)
        n274 = local read "X step size (um)"() -> (w694:dbl)
        n275 = local read "Y step size (um)"() -> (w693:dbl)
        n276 = local read "X0 Position(mm)"() -> (w698:dbl)
        n277 = local read "Y0 Position(mm)"() -> (w697:dbl)
        n278 = local read "X speed (mm/s)"() -> (w692:dbl)
        n279 = local read "X scan distance (mm)"() -> (w696:dbl)
        n280 = local read "Y scan distance (mm)"() -> (w695:dbl)
        n281 = Build Array(w698, w697, w696, w695, w694, w693, w692, w691) -> (w690:dbl[])
        n282 = TDMS Set Properties(5:w690, 7:string[] ["X0 (mm)", "Y0 (mm)", "X scan distance (mm)", "Y scan distance (mm)", "X step size (um)", "Y step size (um)", "X speed (mm/s)", "num of lines"] ("property names"), 8:w701, 10:"Encoder" ("group name"), 11:w702) -> (0:w688:errorcluster, 3:w689:refnum<k34>)  [unwired: 1 in, 2 out]
        n283 = TDMS Close(8:w688, 11:w689) -> (0:w687:errorcluster)  [unwired: 1 out]
        n284 = call <vilib>:"Add State(s) to Queue__JKI_lib_State_Machine.vi"("State(s) in (\"\")"=w709) -> ("States Out"=w708:string)  [unwired: 14 in]
      }
      frame "---------- FLIm ----------" {
        # "Template Separator\n(You can make a copy of, or modify, this frame)"
        n285 = call <vilib>:"Add State(s) to Queue__JKI_lib_State_Machine.vi"("State(s) in (\"\")"=w713) -> ("States Out"=w712:string)  [unwired: 14 in]
      }
      frame "FLIm: remoteStart" {
        # "remote start FLIm\n(You can make a copy of, or modify, this frame)"
        n286 = call "RemoteEventFGV.vi"("Error In"=w714, "Operation (Read)"=enum16{"Read", "Write"}."Read") -> ("Error Out"=w716:errorcluster, "Remote Event out"=w720:T13)  [unwired: 8 in]
        n287 = Unbundle By Name(w720) -> ("remote start event"=w719:refnum<user-event>)
        n288 = Generate User Event(priority (normal)=usereventprio."high priority", user event=w719, event data cluster=FALSE ("event data"), error in=w716) -> (error out=w715:errorcluster)  [unwired: 1 out]
      }
      frame "FLIm: remoteStop" {
        # "remote stop FLIm\n(You can make a copy of, or modify, this frame)"
        n289 = call "RemoteEventFGV.vi"("Error In"=w724, "Operation (Read)"=enum16{"Read", "Write"}."Read") -> ("Error Out"=w726:errorcluster, "Remote Event out"=w729:T13)  [unwired: 8 in]
        n290 = Unbundle By Name(w729) -> ("remote stop event"=w728:refnum<user-event>)
        n291 = Generate User Event(user event=w728, event data cluster=FALSE ("event data"), error in=w726) -> (error out=w725:errorcluster)  [unwired: 1 in, 1 out]
        n292 = call <vilib>:"Add State(s) to Queue__JKI_lib_State_Machine.vi"("State(s) in (\"\")"=w733) -> ("States Out"=w732:string)  [unwired: 14 in]
      }
      frame "---------- Utility ----------" {
        # "Template Separator\n(You can make a copy of, or modify, this frame)"
        n293 = call <vilib>:"Add State(s) to Queue__JKI_lib_State_Machine.vi"("State(s) in (\"\")"=w737) -> ("States Out"=w736:string)  [unwired: 14 in]
      }
      frame "Utility: Dewell" {
        # "Template Separator\n(You can make a copy of, or modify, this frame)"
        n294 = Decimal String To Number(string=w739) -> (number=w738:i32)  [unwired: 2 in, 1 out]
        n295 = Wait (ms)(milliseconds to wait=w738) -> ()  [unwired: 1 out]
        n296 = call <vilib>:"Add State(s) to Queue__JKI_lib_State_Machine.vi"("State(s) in (\"\")"=w743) -> ("States Out"=w742:string)  [unwired: 14 in]
      }
      frame "Utility: StopScanLoop" {
        # "Template Separator\n(You can make a copy of, or modify, this frame)"
        n297 = Generate User Event(user event=w746, event data cluster=FALSE ("event data")) -> ()  [unwired: 2 in, 2 out]
        n298 = call <vilib>:"Add State(s) to Queue__JKI_lib_State_Machine.vi"("State(s) in (\"\")"=w749) -> ("States Out"=w748:string)  [unwired: 14 in]
      }
      frame "Utility: UpdateJogStep" {
        # "Update Jog Step Size\n(You can make a copy of, or modify, this frame)"
        n299 = Bundle By Name(cluster=w750, "JogStep(mm)"="Jog Step (mm)") -> (w751:T10)
      }
      frame "---------- ThorLabsAPI ----------" {
        # "Template Separator\n(You can make a copy of, or modify, this frame)"
        n300 = call <vilib>:"Add State(s) to Queue__JKI_lib_State_Machine.vi"("State(s) in (\"\")"=w758) -> ("States Out"=w757:string)  [unwired: 14 in]
      }
      frame "ThorLabsAPI: BuildDeviceList" {
        # "get connected device list\n(You can make a copy of, or modify, this frame)"
        n301 = constructor class="DeviceManagerCLI"(error in=w759) -> (reference out=w761:refnum<k24>)  [unwired: 2 in, 2 out]
        n302 = invoke class="DeviceManagerCLI" method="BuildDeviceList"(reference=w761) -> (error out=w760:errorcluster)  [unwired: 2 in, 2 out]
        n303 = call <vilib>:"Add State(s) to Queue__JKI_lib_State_Machine.vi"("State(s) in (\"\")"=w764) -> ("States Out"=w763:string)  [unwired: 14 in]
      }
      frame "---------- New Category ----------" {
        # "Template Separator\n(You can make a copy of, or modify, this frame)"
        n304 = call <vilib>:"Add State(s) to Queue__JKI_lib_State_Machine.vi"("State(s) in (\"\")"=w768) -> ("States Out"=w767:string)  [unwired: 14 in]
      }
      frame "New Category: 1" {
        # "Your code here.\n(You can make a copy of, or modify, this frame)"
        n305 = call <vilib>:"Add State(s) to Queue__JKI_lib_State_Machine.vi"("State(s) in (\"\")"=w772) -> ("States Out"=w771:string)  [unwired: 14 in]
      }
      frame "New Category: 2" {
        # "Your code here.\n(You can make a copy of, or modify, this frame)"
        n306 = call <vilib>:"Add State(s) to Queue__JKI_lib_State_Machine.vi"("State(s) in (\"\")"=w776) -> ("States Out"=w775:string)  [unwired: 14 in]
      }
    }
  }
  n307 = while {
    tunnel: w17 -> [w780]
    tunnel: [w778] -> w12
    tunnel: w5 -> [w777]
    stop <- w779 stop-if-true
    n308 = event shown="[2] <StartScan>: User Event" {
      selector: w780 -> [_ _ _]
      dyn-events: [_ _ _] -> w778
      timeout: 30 -> [_ _ _]
      tunnel: [FALSE ("Quit") TRUE ("Quit") _] -> w779
      tunnel: w777 -> [_ _ w786]
      event Timeout {
        n309 = event-data() -> ()  [unwired: 1 in, 3 out]
      }
      event User Event {
        n310 = event-data() -> ()  [unwired: 1 in, 5 out]
      }
      event User Event {
        w788 = 0.0  # Y
        w789 = 0.0  # X
        n311 = event-data() -> ("X"=w785:dbl[], "Y"=w792:dbl[], "Device(Fast)"=w793:refnum<k24>, "Device(Slow)"=w790:refnum<k24>)  [unwired: 1 in, 4 out]
        n312 = Array Size(array=w785) -> (size(s)=w784:i32)
        n313 = for {
          tunnel: w793 -> [w813]
          tunnel: w785 -> [w804] mode=indexing
          tunnel: w792 -> [w803] mode=indexing
          shift-right: [w809] -> w787
          shift-left: errorcluster {"status"=FALSE, "code"=0, "source"=""} ("error constant") -> [w812]
          tunnel: w790 -> [w811]
          shift-right: [w804] -> _
          shift-left: w789 -> [w807]
          shift-right: [w803] -> _
          shift-left: w788 -> [w806]
          tunnel: w784 -> [w799]
          i -> [w798]
          n314 = Increment(x=w798) -> (x+1=w797:i32)
          n315 = Not Equal?(x=w807, y=w804) -> (x != y?=w808:bool)
          n316 = Not Equal?(x=w803, y=w806) -> (x != y?=w805:bool)
          n317 = Divide(x=w797, y=w799) -> (x/y=w802:dbl)
          n318 = case shown="True" w808 {
            tunnel: w813 -> [_ w829]
            tunnel: w812 -> [w822 w828]
            tunnel: [w822 w825] -> w810
            tunnel: w804 -> [_ w824]
            frame False {
              # "if same x, do nothing"
            }
            frame True {
              # "if different x, move"
              n319 = invoke class="KCubeBrushlessMotor" method="SetMoveAbsolutePosition"(reference=w829, error in=w828, "position"=w824) -> (reference out=w827:refnum<k24>, error out=w826:errorcluster)  [unwired: 1 in, 2 out]
              n320 = invoke class="KCubeBrushlessMotor" method="MoveAbsolute"(reference=w827, error in=w826, "waitTimeout"=10000) -> (error out=w825:errorcluster)  [unwired: 1 in, 3 out]
            }
          }
          n321 = Multiply(x=100.0, y=w802) -> (x*y=→"Scan Progress":dbl)
          n322 = case shown="True" w805 {
            tunnel: w811 -> [_ w821]
            tunnel: w810 -> [w814 w820]
            tunnel: [w814 w817] -> w809
            tunnel: w803 -> [_ w816]
            frame False {
              # "If same y, do nothing"
            }
            frame True {
              # "if different y, move"
              n323 = invoke class="KCubeDCServo" method="SetMoveAbsolutePosition"(reference=w821, error in=w820, "position"=w816) -> (reference out=w819:refnum<k24>, error out=w818:errorcluster)  [unwired: 1 in, 2 out]
              n324 = invoke class="KCubeDCServo" method="MoveAbsolute"(reference=w819, error in=w818, "waitTimeout"=10000) -> (error out=w817:errorcluster)  [unwired: 1 in, 3 out]
            }
          }
        }
        n325 = call <vilib>:"Simple Error Handler.vi"("error in (no error)"=w787) -> ()  [unwired: 4 in, 5 out]
        n326 = flat-sequence {
          tunnel: w787 -> [_]
          tunnel: w786 -> [w796]
          frame #0 {
            n327 = Generate User Event(priority (normal)=usereventprio."high priority", user event=w796, event data cluster=FALSE ("event data")) -> ()  [unwired: 1 in, 2 out]
          }
        }
      }
    }
  }
  n328 = Destroy User Event(user event=w5, error in=w6) -> (error out=w7:errorcluster)
  n329 = Destroy User Event(user event=w11, error in=w7) -> (error out=w9:errorcluster)
  n330 = Destroy User Event(user event=w10, error in=w9) -> (error out=w8:errorcluster)
  n331 = Unregister For Events(event registration refnum=w12, error in=w8) -> (error out=w3:errorcluster)
  n332 = Unregister For Events(event registration refnum=w2, error in=w3) -> (error out=→"error out":errorcluster)
